vi "IO_Process.vi"(8 "error in":errorcluster, 10 "TopLevel":refnum<class "TopLevel.lvclass">, 11 "IO in":refnum<class "IO.lvclass">) -> (3 "IO out":refnum<class "IO.lvclass">)   [LabVIEW 2022 SP3, in "IO.lvclass"]
uses:
  IO.lvclass
  TopLevel/TopLevel.lvclass
  TopLevel/Typedefs/Digilens Config Cluster.ctl
  TopLevel/Typedefs/Motor Controller Config Data.ctl
  Typedefs/IO Config Data.ctl
  Typedefs/DCON_DeviceConfig--Cluster.ctl
  Typedefs/Channel Data.ctl
  GIS Printer/Typedefs/PrinterConfiguration--Cluster.ctl
  DAQWFE/LV_Source/Subsystems/DAQ/DataTypes/TD DAQ Settings--cluster.ctl
  DAQWFE/LV_Source/Subsystems/DAQ/DataTypes/TD DI Instrument Settings--cluster.ctl
  DAQWFE/LV_Source/Subsystems/DAQ/DataTypes/TD AI Instrument Settings--cluster.ctl
  DAQWFE/LV_Source/Subsystems/DAQ/DataTypes/TD AI InstSettings--cluster.ctl
  DAQWFE/LV_Source/Subsystems/DAQ/Process/ProcessSupport/TD SimAI Ranges--cluster.ctl
  Typedefs/ReadbackQuery--Cluster.ctl
  Typedefs/Device Names.ctl
  Typedefs/DCON Action Engine-States.ctl
  Typedefs/DO Value API Data.ctl
  Typedefs/AO Value API Data.ctl
  Typedefs/API Event Data.ctl
  Typedefs/API Task State.ctl
  Typedefs/API Command Cluster.ctl
  Typedefs/API Command Enum.ctl
  Typedefs/Purge PH API Data.ctl
  Typedefs/ICP1-D0 Channel Names.ctl
  Typedefs/ICP2-DI Channel Names.ctl
  Typedefs/ICP2-DO Channel Names.ctl
  Typedefs/ICP1-AI Channel Names.ctl
  Typedefs/ICP1-AO Channel Names.ctl
  Typedefs/ICP2-AO Channel Names.ctl
  Motor Controller/Motor Controller.lvclass
  GIS Printer/GIS Printer.lvclass
  DAQWFE/LV_Source/Subsystems/DAQ/DAQ.lvclass
panel:
  out "error out":errorcluster
  in  "OK":bool
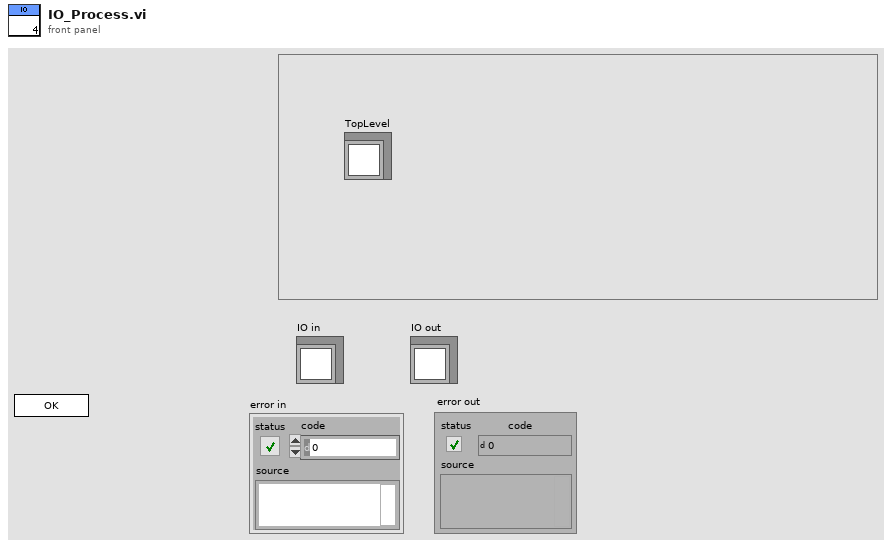
[diagram p1: front panel]
types:
  T1 = typedef "ReadbackQuery--Cluster.ctl" = cluster{"Device Name":T2, "Action":T3}
  T2 = typedef "IO.lvclass/Device Names.ctl" = enum16{"ICP1-DO", "ICP2-DI", "ICP2-DO", "ICP1-AI", "ICP1-AO", "ICP2-AO"}
  T3 = typedef "DCON Action Engine-States.ctl" = enum16{"Open", "Close", "Set DO Value", "Get Digital Status", "Get Data", "Get AI Status", "Set AO Value", "Get AO Status"}
  T4 = typedef "TopLevel.lvclass/Digilens Config Cluster.ctl" = cluster{"Motion Controller":T5, "IO Config":T6, "PrinterConfiguration":T9, "DAQ Settings":T10}
  T5 = typedef "Motor Controller.lvclass/Motor Controller Config Data.ctl" = cluster{"Motor IP Addresss":string, "Current Position":i32, "Pulse_Per_mm":i32, "PrePrint":dbl[], "Load Position_mm":i32, "Laminate Position_mm":i32}
  T6 = typedef "IO.lvclass/IO Config Data.ctl" = cluster{"DAQDevices":T7[], "DI Channels":T8[], "DO Channels":T8[], "Material Names":string[], "AI Channels":T8[], "AO Channels":T8[]}
  T7 = typedef "IO.lvclass/DCON_DeviceConfig--Cluster.ctl" = cluster{"COM":string, "DeviceName":string, "BaudRate":u32, "Number of Channels":i32, "DeviceAddress":i32, "Enable":bool}
  T8 = typedef "IO.lvclass/Channel Data.ctl" = cluster{"Channel Name":string, "Device Name":string, "Channel No":string}
  T9 = typedef "GIS Printer.lvclass/PrinterConfiguration--Cluster.ctl" = cluster{"IPAddress":string, "Move Stage on RTP Command?":bool, "Stage Move Position":string, "PH1-Prime Path":path, "PH2-Prime Path":path, "PH3-Prime Path":path, "PH4-Prime Path":path, "PH5-Prime Path":path, "PH6-Prime Path":path, "PrintScriptsFolder":path, "PurgeScriptsFolder":path, "StageScriptsFolder":path, "PH1-HeatOn Path":path, "PH2-HeatOn Path":path, "PH3-HeatOn Path":path, "PH4-HeatOn Path":path, "PH5-HeatOn Path":path, "PH6-HeatOn Path":path, "PH1-HeatOff Path":path, "PH2-HeatOff Path":path, "PH3-HeatOff Path":path, "PH4-HeatOff Path":path, "PH5-HeatOff Path":path, "PH6-HeatOff Path":path}
  T10 = typedef "DAQ.lvclass/TD DAQ Settings--cluster.ctl" = cluster{"Simulate DAQ":bool, "DI Settings":T11[], "AI Settings":T12[], "Relay IONames":string[], "AO IONames":string[], "AO NChan SingleTask":bool}
  T11 = typedef "DAQ.lvclass/TD DI Instrument Settings--cluster.ctl" = cluster{"Disable":bool, "DI TaskName":string, "DI RefreshIntv":i32}
  T12 = typedef "DAQ.lvclass/TD AI Instrument Settings--cluster.ctl" = cluster{"Disable":bool, "AI TaskName":string, "AI InstSettings":T13, "SimAI Ranges":T14}
  T13 = typedef "DAQ.lvclass/TD AI InstSettings--cluster.ctl" = cluster{"DaqRate":dbl, "NumSamples":i32}
  T14 = typedef "DAQ.lvclass/TD SimAI Ranges--cluster.ctl" = cluster{"lo":dbl, "hi":dbl}
  T15 = cluster{"IOLoopEvents":refnum<user-event>, "Open":bool, "Digilens Config":T4}
  T16 = typedef "IO.lvclass/API Event Data.ctl" = cluster{"Task":cluster{"Time Stamp":timestamp, "Timeout (ms)":u32, "Task State":T17, "Task Error":errorcluster, "Task ID":string}, "Command":variant, "Return Value":variant}
  T17 = typedef "IO.lvclass/API Task State.ctl" = enum16{"Completed", "Errored", "Pending"}
  T18 = typedef "IO.lvclass/API Command Cluster.ctl" = cluster{"Command":T19, "Arguments":string, "Data":variant}
  T19 = typedef "IO.lvclass/API Command Enum.ctl" = enum16{"Set DO Value", "Set AO Value", "Purge PH"}
  T20 = enum32{"invalid app kind", "Development System", "Run Time System", "Student Edition", "Embedded LabVIEW", "Evaluation", "Custom"}
  T21 = enum32{"Invalid", "Standard", "Closed", "Hidden", "Minimized", "Maximized"}
  T22 = typedef "IO.lvclass/DO Value API Data.ctl" = cluster{"Device Name":T2, "Value":bool, "Index":i32}
  T23 = typedef "IO.lvclass/AO Value API Data.ctl" = cluster{"Device Name":T2, "Index":i32, "Value":dbl}
  T24 = typedef "IO.lvclass/Purge PH API Data.ctl" = cluster{"ICP1-DO Channel Name":T25, "Duration (s)":dbl}
  T25 = typedef "IO.lvclass/ICP1-D0 Channel Names.ctl" = enum16{"None", "Meniscus Pressure Reg PWR - R1", "Meniscus Pressure Reg PWR - R2", "Meniscus Pressure Reg PWR - R3", "Meniscus Pressure Reg PWR - R4", "Meniscus Pressure Reg PWR - R5", "Meniscus Pressure Reg PWR - R6", "Clear Stage Alarm", "Servo ON", "Purge Valve Open - R1", "Purge Valve Open - R2", "Purge Valve Open - R3", "Purge Valve Open - R4", "Purge Valve Open - R5", "Purge Valve Open - R6"}
  T26 = typedef "IO.lvclass/ICP2-DI Channel Names.ctl" = enum16{"None", "SW - Ink Valve - R1", "SW - Ink Valve - R2", "SW - Ink Valve - R3", "SW - Ink Valve - R4", "SW - Ink Valve - R5", "SW - Ink Valve - R6", "SW - COVER INPUT SIDE", "SW - COVER OUTPUT SIDE", "SW - Purge - R1", "SW - Purge - R2", "SW - Purge - R3", "SW - Purge - R4", "SW - Purge - R5", "SW - Purge - R6"}
  T27 = typedef "IO.lvclass/ICP2-DO Channel Names.ctl" = enum16{"None", "Meniscus Valve Open - R1", "Meniscus Valve Open - R2", "Meniscus Valve Open - R3", "Meniscus Valve Open - R4", "Meniscus Valve Open - R5", "Meniscus Valve Open - R6", "Ink Flow Valve Open - R1", "Ink Flow Valve Open - R2", "Ink Flow Valve Open - R3", "Ink Flow Valve Open - R4", "Ink Flow Valve Open - R5", "Ink Flow Valve Open - R6", "SW_LED - Ink Valve - R1", "SW_LED - Ink Valve - R2", "SW_LED - Ink Valve - R3", "Recirc Pump On - R1", "Recirc Pump On - R2", "Recirc Pump On - R3", "Recirc Pump On - R4", "Recirc Pump On - R5", "Recirc Pump On - R6", "SW_LED - Ink Valve - R4", "SW_LED - Ink Valve - R5", "SW_LED - Ink Valve - R6"}
  T28 = typedef "IO.lvclass/ICP1-AI Channel Names.ctl" = enum16{"None", "Meniscus Pressure Read - R1", "Meniscus Pressure Read - R2", "Meniscus Pressure Read - R3", "Meniscus Pressure Read - R4", "Meniscus Pressure Read - R5", "Meniscus Pressure Read - R6", "Meniscus Pressure Set - R1", "Meniscus Pressure Set - R2", "Meniscus Pressure Set - R3", "Meniscus Pressure Set - R4", "Meniscus Pressure Set - R5", "Meniscus Pressure Set - R6"}
  T29 = typedef "IO.lvclass/ICP1-AO Channel Names.ctl" = enum16{"None", "Meniscus Pressure Set - R1", "Meniscus Pressure Set - R2", "Meniscus Pressure Set - R3", "Meniscus Pressure Set - R4", "Meniscus Pressure Set - R5", "Meniscus Pressure Set - R6", "Meniscus Vac Pump Speed"}
  T30 = typedef "IO.lvclass/ICP2-AO Channel Names.ctl" = enum16{"None", "Recirc Pump Flow Set - R1", "Recirc Pump Flow Set - R2", "Recirc Pump Flow Set - R3", "Recirc Pump Flow Set - R4", "Recirc Pump Flow Set - R5", "Recirc Pump Flow Set - R6"}
  T31 = cluster{"Time Stamp":timestamp, "Timeout (ms)":u32, "Task State":T17, "Task Error":errorcluster, "Task ID":string}
  T32 = cluster{"Core":cluster{"Current VI Reference":refnum<vi>, "Close Panel on Exit?":bool}, "TopLevel out":refnum<class "IO.lvclass">, "Tasks":T16[], "TO":i32, "API Executed Event":refnum<user-event>, "API Return Event":refnum<user-event>, "Task Start ms":u32, "Current Task. Return Value":variant, "Methods:Accessors:Digilens Config":T4, "Current Task":T18, "DCONOpen":bool}
  T33 = cluster{"Current VI Reference":refnum<vi>, "Close Panel on Exit?":bool}
  T34 = typedef "IO.lvclass/UserEvents.ctl" = cluster{"API Incoming Event":refnum<user-event>, "API Executed Event":refnum<user-event>, "API Return Event":refnum<user-event>, "Status Changed Event":refnum<user-event>}
  T35 = typedef "TopLevel.lvclass/UserEvents.ctl" = cluster{"API Incoming Event":refnum<user-event>, "API Executed Event":refnum<user-event>, "API Return Event":refnum<user-event>, "Exit Event":refnum<user-event>, "StatusChanged":refnum<user-event>, "DLP GUI Config Changed":refnum<user-event>, "AppEvent":refnum<user-event>, "Login Event":refnum<user-event>, "HeadPrimeStatusEvent":refnum<user-event>}
  T36 = typedef "IO.lvclass/DCON Private Data.ctl" = cluster{"DeviceName":string, "Number of Channels":i32, "COM":refnum<visa-resource-name>, "Status String":string, "Input String":string, "Value ":i32, "Digital Bits Value":bool[], "Analog Values":dbl[], "DeviceAddress":i32, "Enable":bool}
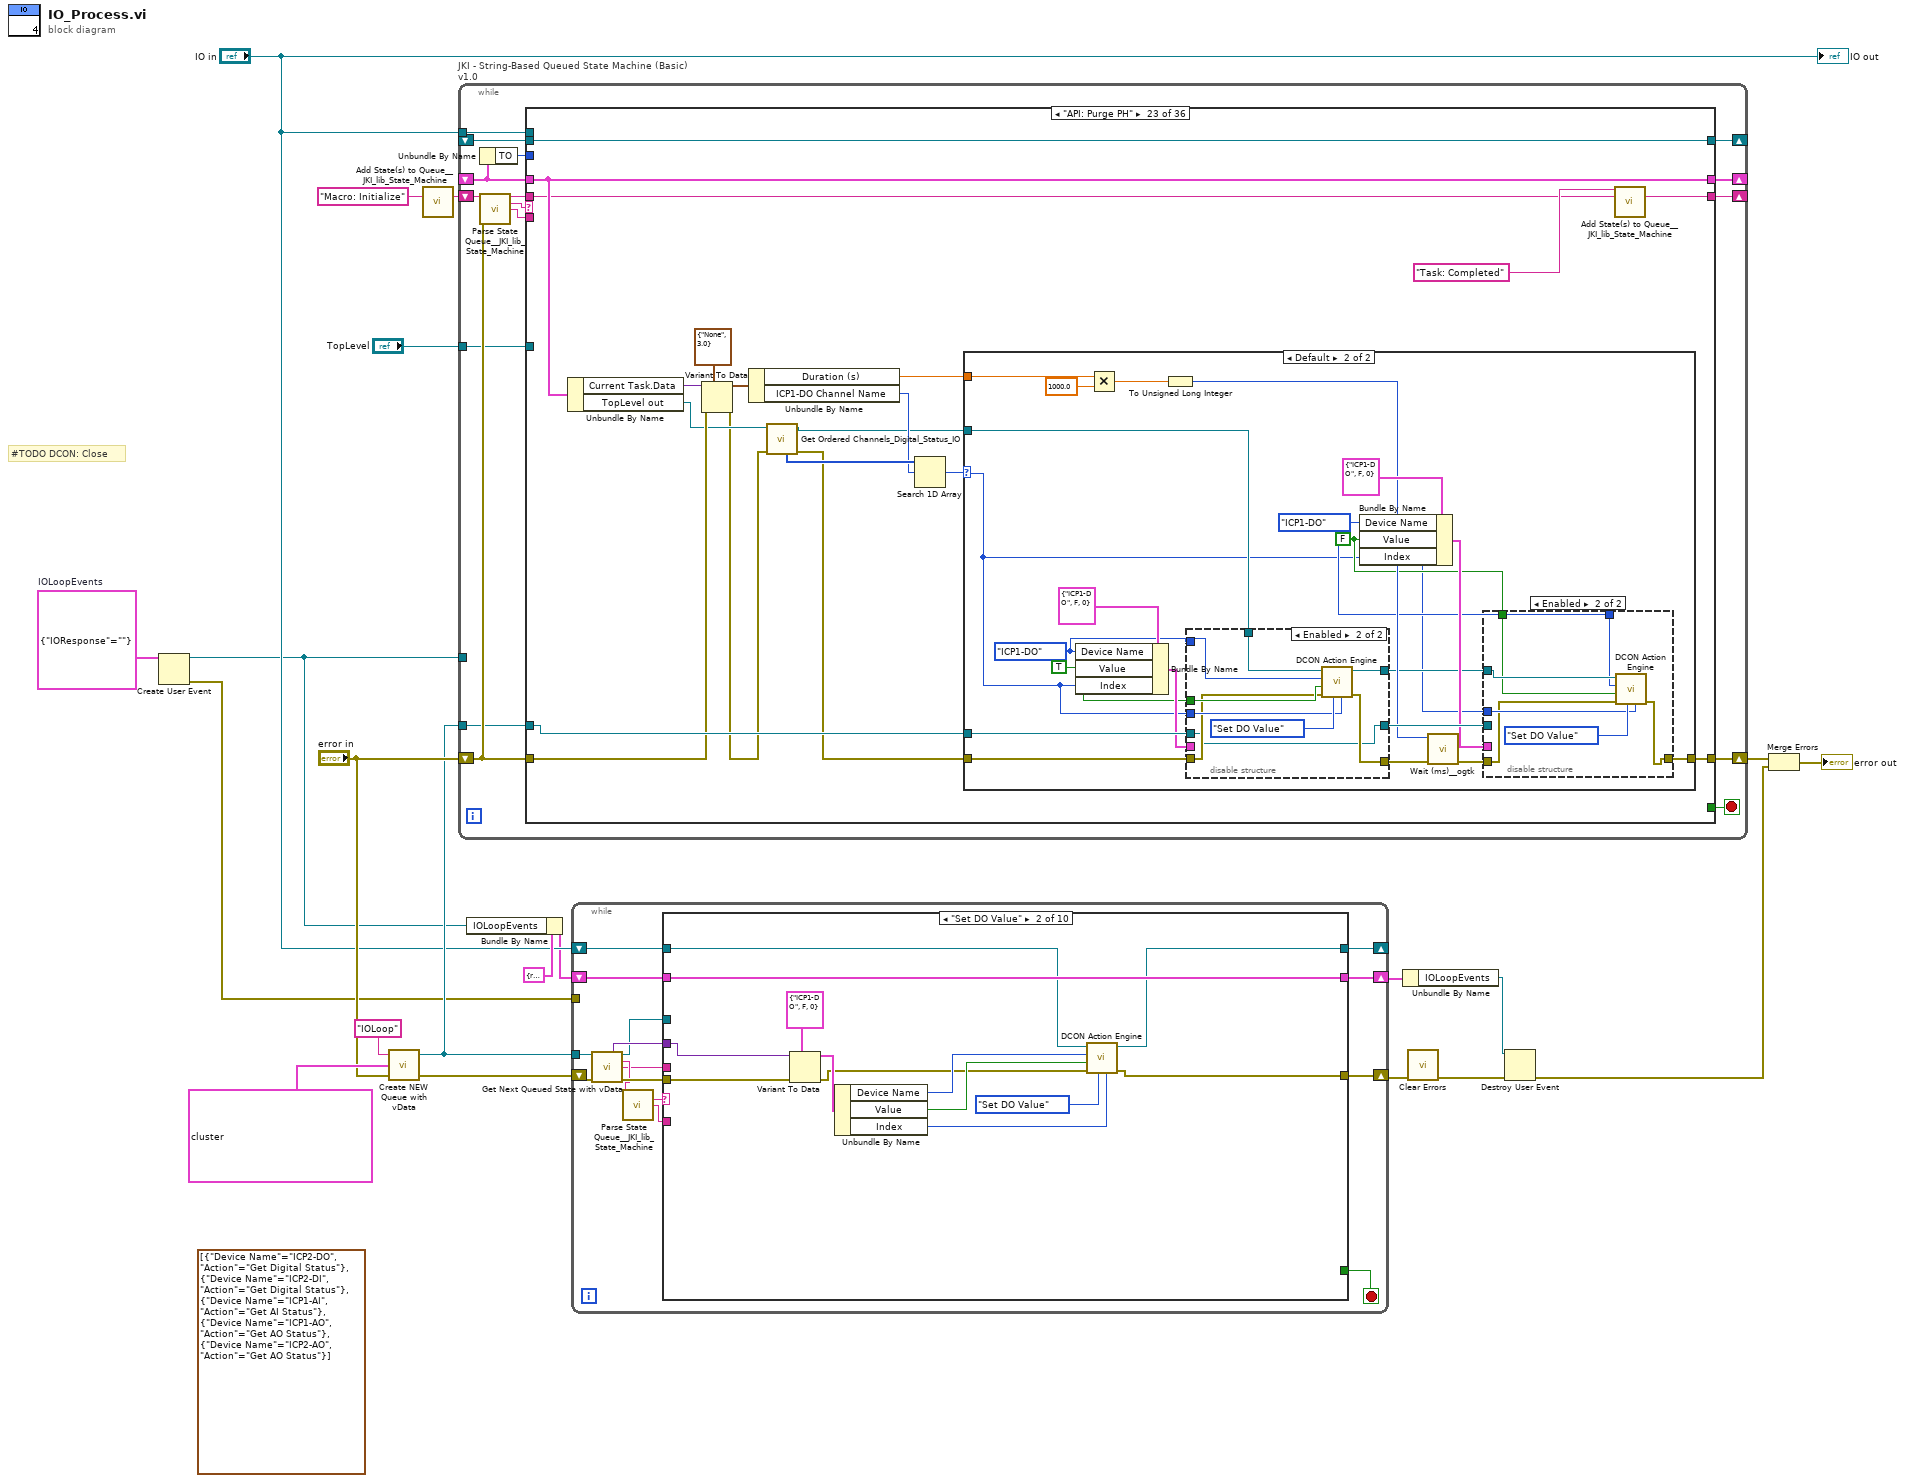
[diagram p0: block diagram]
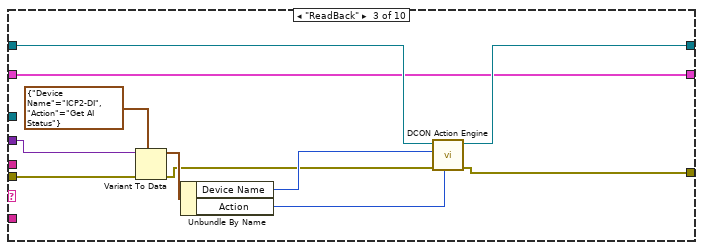
[diagram p3: hidden frame]
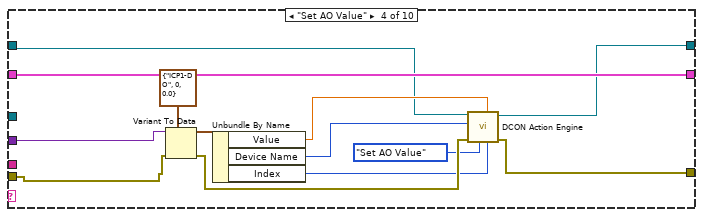
[diagram p4: hidden frame]
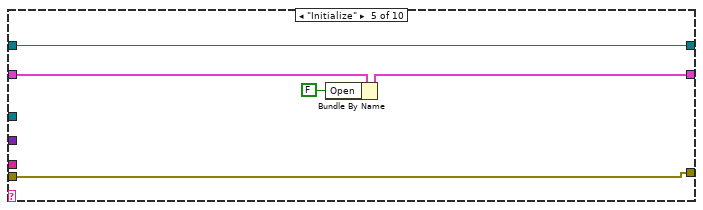
[diagram p5: hidden frame]
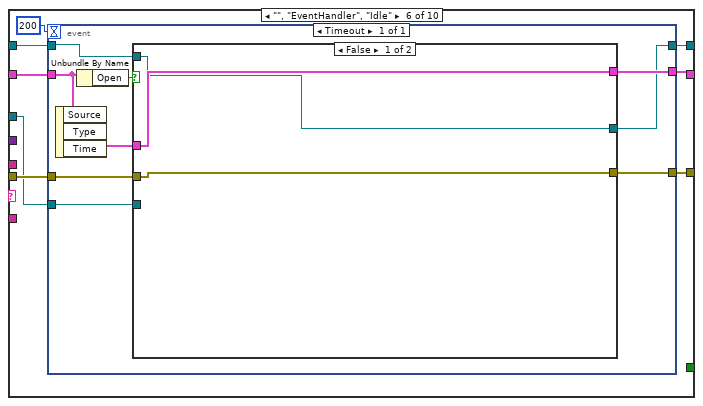
[diagram p6: hidden frame]
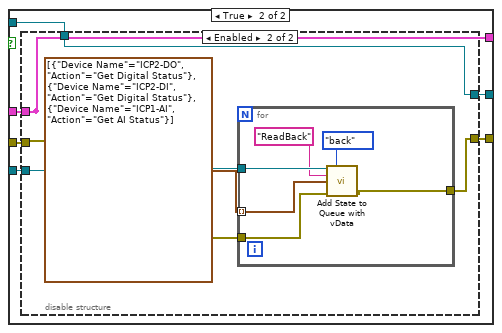
[diagram p7: hidden frame]
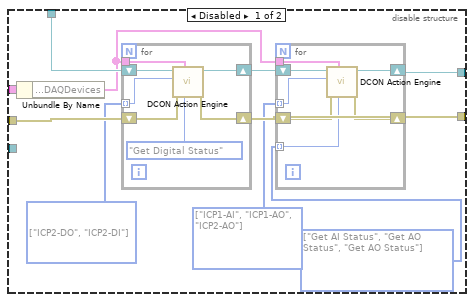
[diagram p8: hidden frame]
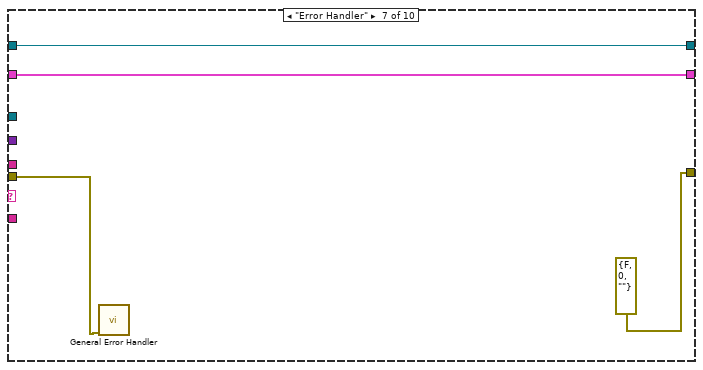
[diagram p9: hidden frame]
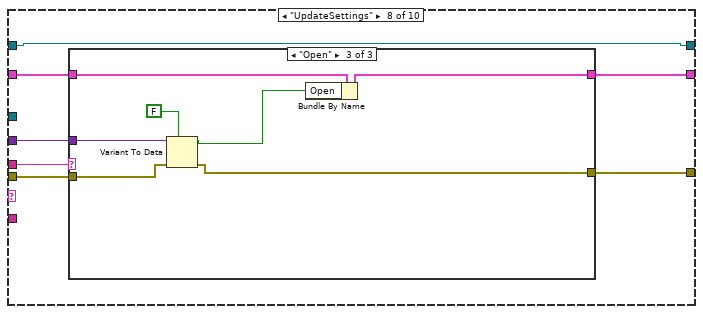
[diagram p10: hidden frame]
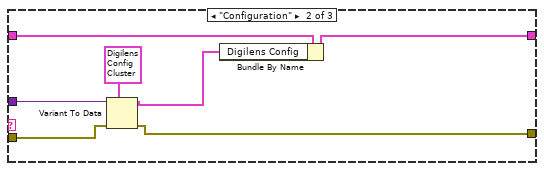
[diagram p12: hidden frame]
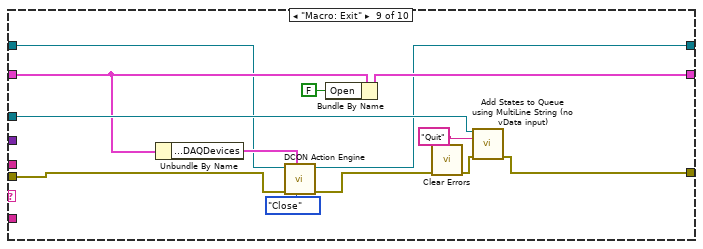
[diagram p13: hidden frame]
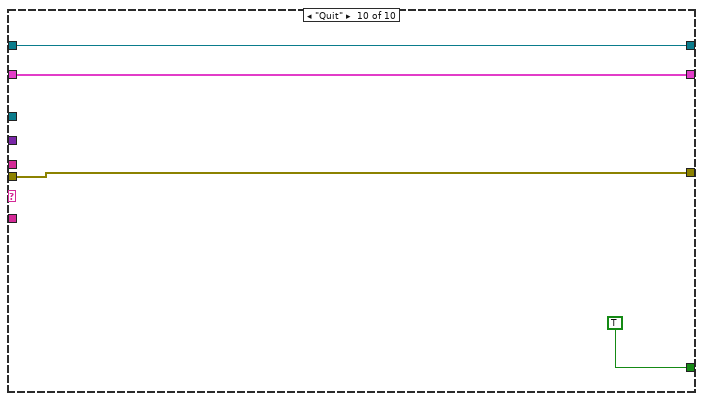
[diagram p14: hidden frame]
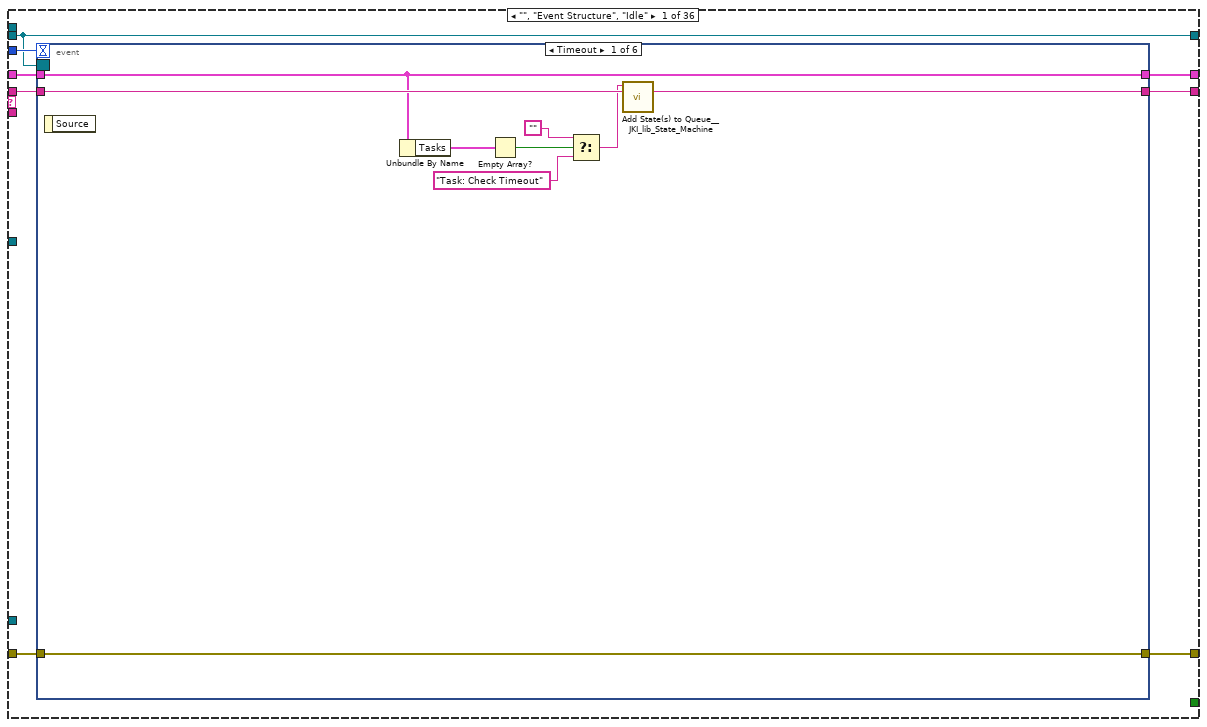
[diagram p15: hidden frame]
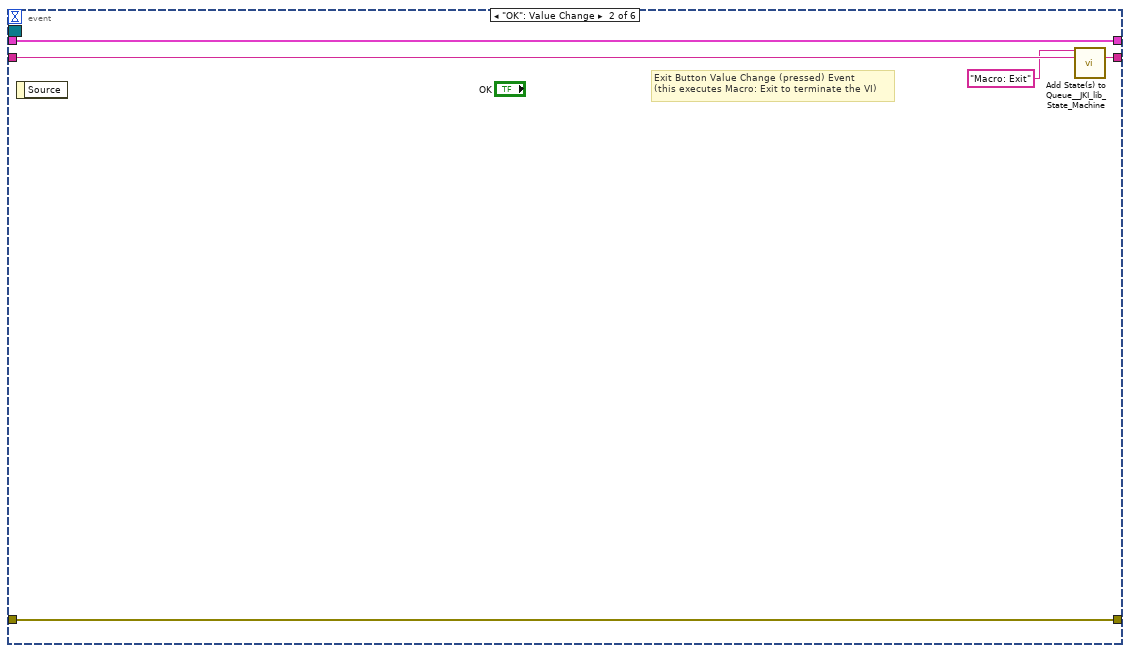
[diagram p16: hidden frame]
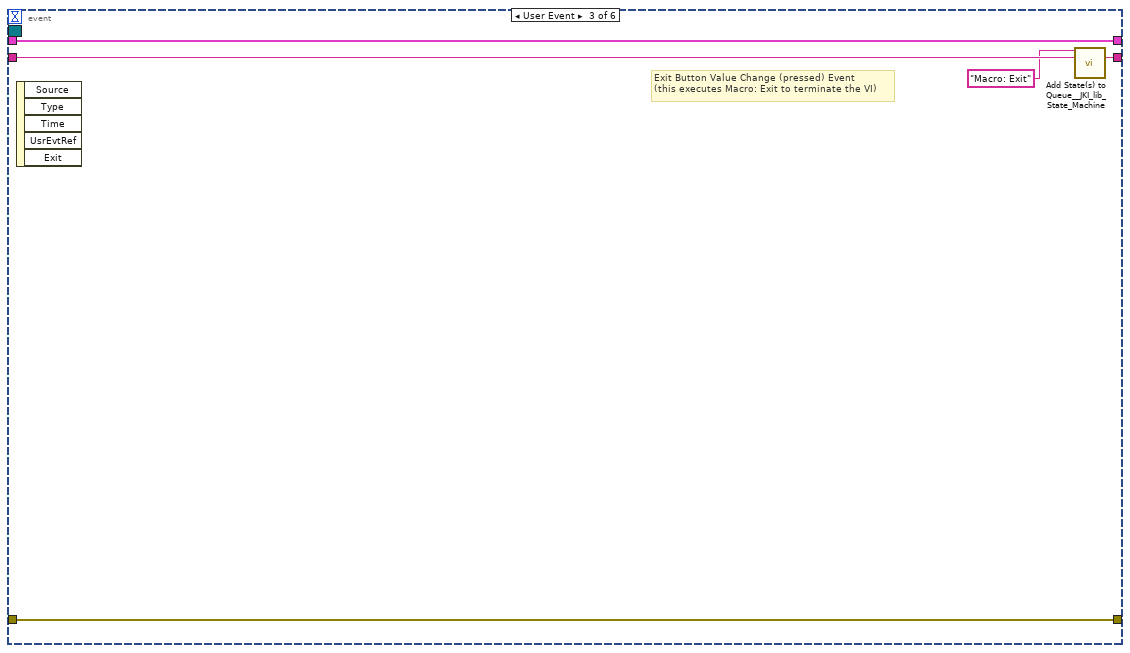
[diagram p17: hidden frame]
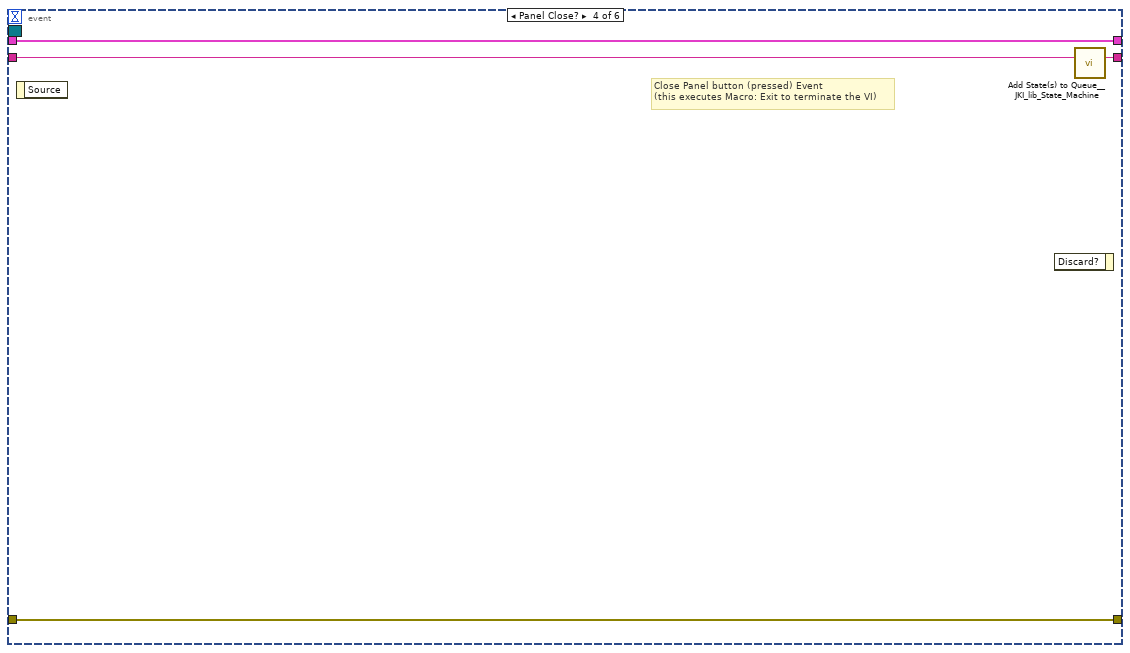
[diagram p18: hidden frame]
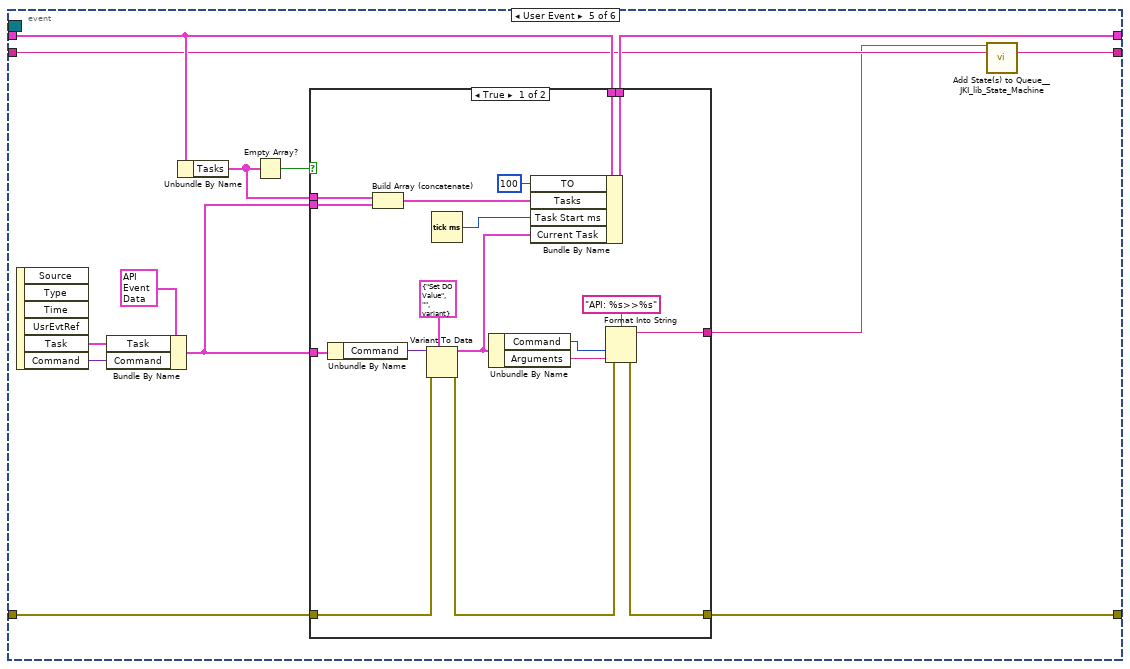
[diagram p19: hidden frame]
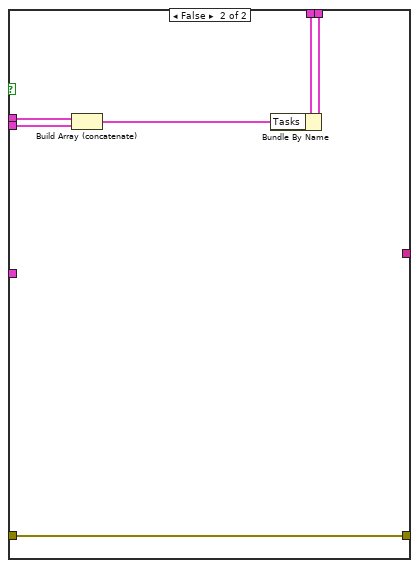
[diagram p20: hidden frame]
diagram:
  (unwired) T1[] [{"Device Name"=enum."ICP2-DO", "Action"=enum."Get Digital Status"}, {"Device Name"=enum."ICP2-DI", "Action"=enum."Get Digital Status"}, {"Device Name"=enum."ICP1-AI", "Action"=enum."Get AI Status"}, {"Device Name"=enum."ICP1-AO", "Action"=enum."Get AO Status"}, {"Device Name"=enum."ICP2-AO", "Action"=enum."Get AO Status"}]
  w17 = cluster{"IOResponse":string} {"IOResponse"=""}  # IOLoopEvents
  # "#TODO DCON: Close"
  n1 = Create User Event(user event datatype=w17) -> (user event=w5:refnum<user-event>, error out=w8:errorcluster)  [unwired: 1 in]
  n2 = call <vilib>:"Create NEW Queue with vData.vi"("error in (no error)"="error in", "Initial States"=cluster{"state":string, "vData":variant}[] [{"state"="Initialize", "vData"=variant}, {"state"="Idle", "vData"=variant}], "Name (SMQ)"="IOLoop") -> ("error out"=w12:errorcluster, "queue out"=w11:refnum<queue>)  [unwired: 1 in]
  n3 = call <vilib>:"Add State(s) to Queue__JKI_lib_State_Machine.vi"("State(s) in (\"\")"="Macro: Initialize") -> ("States Out"=w21:string)  [unwired: 14 in]
  n4 = while "JKI - String-Based Queued State Machine (Basic) v1.0" {
    shift-right: [w30] -> _
    shift-left: _ -> [w24]
    shift-right: [w33] -> w19
    shift-left: "error in" -> [w29]
    shift-right: [w32] -> _
    shift-left: w21 -> [w34]
    tunnel: "IO in" -> [w28]
    shift-right: [w27] -> _
    shift-left: _ -> [w26]
    tunnel: "TopLevel" -> [w23]
    tunnel: w5 -> [_]
    tunnel: w11 -> [w22]
    stop <- w31 stop-if-true
    n5 = Unbundle By Name(w24) -> ("TO"=w25:i32)
    n6 = call <vilib>:"Parse State Queue__JKI_lib_State_Machine.vi"("State Queue"=w34, "Error In (no error)"=w29) -> ("Remaining States"=w36:string, "Current State"=w37:string, "Arguments"=w35:string)  [unwired: 11 in]
    n7 = case shown="\"API: Purge PH\"" w37 {
      selector: w37 -> [_ _ w148 _ _ _ _ _ _ _ _ _ _ _ _ _ _ _ _ _ _ _ _ _ _ _ _ _ _ _ _ _ _ _ _ _]
      tunnel: w36 -> [w45 w146 w152 w171 w178 w184 w189 w213 w220 w225 w231 w238 w250 w277 _ w298 w309 w323 w329 w331 w339 w370 w403 w460 w471 w490 w511 w546 w558 w571 w583 w627 w671 w715 w759 w803]
      tunnel: w35 -> [_ _ _ _ _ _ _ _ _ _ _ w233 w244 _ _ _ _ _ _ _ _ _ _ _ _ _ _ _ _ _ _ _ _ _ _ _]
      tunnel: w24 -> [w43 w143 w150 w162 w175 w182 w186 _ w215 w222 w229 w236 w246 w274 w279 w296 w307 w320 w327 w332 w343 w375 w406 w461 w469 w488 w508 w543 w557 w569 w581 w625 w669 w713 w757 w801]
      tunnel: [w42 w144 w154 w168 errorcluster {"status"=FALSE, "code"=0, "source"=""} ("error out") w181 w187 w195 w216 w223 w226 w234 w247 w275 w282 w288 w308 w318 w326 w330 w335 w367 w402 w459 w465 w485 w516 w542 w559 w564 w579 w623 w667 w711 w755 w799] -> w33
      tunnel: w29 -> [w41 w144 w153 w168 w174 w181 w187 w206 w217 w223 w227 w235 w248 w275 w282 w283 w308 w311 w325 w330 w342 w374 w396 w459 w464 w484 w515 w541 w559 w567 w578 w622 w666 w710 w754 w798]
      tunnel: [w44 w145 w151 w170 w177 w183 w188 w212 w219 w224 w230 w237 w249 w276 w281 w297 w309 w322 w328 w331 w340 w371 w404 w460 w471 w490 w512 w547 w558 w571 w583 w627 w671 w715 w759 w803] -> w32
      tunnel: [_ _ _ _ _ TRUE _ _ _ _ _ _ _ _ _ _ _ _ _ _ _ _ _ _ _ _ _ _ _ _ _ _ _ _ _ _] -> w31
      tunnel: [w40 w143 w150 w169 w175 w182 w186 w211 w215 w222 w229 w236 w246 w274 w279 w296 w307 w320 w327 w332 w343 w375 w406 w461 w469 w488 w509 w540 w557 w562 w581 w625 w669 w713 w757 w801] -> w30
      tunnel: w25 -> [w39 _ _ _ _ _ _ _ _ _ _ _ _ _ _ _ _ _ _ _ _ _ _ _ _ _ _ _ _ _ _ _ _ _ _ _]
      tunnel: w28 -> [_ _ _ _ _ _ _ w191 _ _ _ _ _ _ _ _ _ _ _ _ _ _ _ _ _ _ _ _ _ _ _ _ _ _ _ _]
      tunnel: [w38 w142 w147 w159 w172 w179 w185 w209 w214 w221 w228 w232 w243 w273 w278 w293 w306 w321 w324 w333 w344 w376 w407 w462 w470 w489 w519 w548 w556 w570 w582 w626 w670 w714 w758 w802] -> w27
      tunnel: w26 -> [w38 w142 w147 w159 w172 w179 w185 w209 w214 w221 w228 w232 w243 w273 w278 w293 w306 _ w324 w333 w344 w376 w407 w462 w470 w489 w519 w548 w556 w570 w582 w626 w670 w714 w758 w802]
      tunnel: w23 -> [_ _ _ _ _ _ _ w200 _ _ _ _ _ _ _ _ _ w313 _ _ _ _ _ _ _ _ _ _ _ _ _ _ _ _ _ _]
      tunnel: w22 -> [_ _ _ _ _ _ _ w193 _ _ _ _ _ _ _ w285 _ _ _ _ w337 w366 w401 _ _ _ _ _ _ w563 _ _ _ _ _ _]
      frame "", "Event Structure", "Idle" {
        n8 = event shown="[0] Timeout" {
          selector: w38 -> [_ _ _ _ _ _]
          dyn-events: _ -> [_ _ _ _ _ _]
          timeout: w39 -> [_ _ _ _ _ _]
          tunnel: w45 -> [w54 w59 w64 w68 w70 w125]
          tunnel: [w53 w58 w63 w67 w71 w126] -> w44
          tunnel: w43 -> [w51 w56 w61 w65 w75 w124]
          tunnel: [w52 w57 w62 w66 w73 w118] -> w42
          tunnel: w41 -> [w52 w57 w62 w66 w72 w119]
          tunnel: [w51 w56 w61 w65 w76 w121] -> w40
          event Timeout {
            n9 = event-data() -> ()  [unwired: 1 in, 1 out]
            n10 = Unbundle By Name(w51) -> ("Tasks"=w50:T16[])
            n11 = Empty Array?(array=w50) -> (empty?=w49:bool)
            n12 = Select(t="", s=w49, f="Task: Check Timeout") -> (s? t:f=w46:string)
            n13 = call <vilib>:"Add State(s) to Queue__JKI_lib_State_Machine.vi"("State(s) in Front (\"\")"=w46, "State(s) in (\"\")"=w54) -> ("States Out"=w53:string)  [unwired: 13 in]
          }
          event "OK": Value Change {
            # "Exit Button Value Change (pressed) Event\n(this executes Macro: Exit to terminate the VI)"
            n14 = event-data() -> ()  [unwired: 1 in, 1 out]
            n15 = call <vilib>:"Add State(s) to Queue__JKI_lib_State_Machine.vi"("State(s) in Front (\"\")"="Macro: Exit", "State(s) in (\"\")"=w59) -> ("States Out"=w58:string)  [unwired: 13 in]
          }
          event User Event {
            # "Exit Button Value Change (pressed) Event\n(this executes Macro: Exit to terminate the VI)"
            n16 = event-data() -> ()  [unwired: 1 in, 5 out]
            n17 = call <vilib>:"Add State(s) to Queue__JKI_lib_State_Machine.vi"("State(s) in Front (\"\")"="Macro: Exit", "State(s) in (\"\")"=w64) -> ("States Out"=w63:string)  [unwired: 13 in]
          }
          event Panel Close? {
            # "Close Panel button (pressed) Event\n(this executes Macro: Exit to terminate the VI)"
            n18 = event-data() -> ()  [unwired: 1 in, 1 out]
            n19 = event-data() -> ()  [unwired: 2 in, 1 out]
            n20 = call <vilib>:"Add State(s) to Queue__JKI_lib_State_Machine.vi"("State(s) in (\"\")"=w68) -> ("States Out"=w67:string)  [unwired: 14 in]
          }
          event User Event {
            n21 = event-data() -> ("Task"=w80:T31, "Command"=w79:variant)  [unwired: 1 in, 4 out]
            n22 = Bundle By Name(cluster=T16 {"Task"={"Time Stamp"=timestamp(0 s since 1904-01-01), "Timeout (ms)"=0, "Task State"=enum."Completed", "Task Error"={"status"=FALSE, "code"=0, "source"=""}, "Task ID"=""}, "Command"=variant, "Return Value"=variant} ("API Event Data"), "Task"=w80, "Command"=w79) -> (w74:T16)
            n23 = Unbundle By Name(w75) -> ("Tasks"=w77:T16[])
            n24 = Empty Array?(array=w77) -> (empty?=w78:bool)
            n25 = case shown="True" w78 {
              tunnel: w77 -> [w99 w105]
              tunnel: w74 -> [w98 w104]
              tunnel: w75 -> [w97 w103]
              tunnel: [w95 w101] -> w76
              tunnel: w74 -> [w94 _]
              tunnel: w72 -> [w91 w100]
              tunnel: [w89 w100] -> w73
              tunnel: [w86 _] -> w69
              frame True {
                n26 = Unbundle By Name(w94) -> ("Command"=w93:variant)
                n27 = Build Array (concatenate)(w99, w98) -> (w96:T16[])
                n28 = Variant To Data(error in=w91, type=T18 {"Command"=enum."Set DO Value", "Arguments"="", "Data"=variant} ("API Command Cluster"), Variant=w93) -> (data=w82:T18, error out=w90:errorcluster)
                n29 = Tick Count (ms)() -> (millisecond timer value=w84:u32)
                n30 = Unbundle By Name(w82) -> ("Command"=w87:T19, "Arguments"=w85:string)
                n31 = Bundle By Name(cluster=w97, "TO"=100, "Tasks"=w96, "Task Start ms"=w84, "Current Task"=w82) -> (w95:T32)
                n32 = Format Into String(format string="API: %s>>%s", error in=w90, w87, w85) -> (resulting string=w86:string, error out=w89:errorcluster)  [unwired: 1 in]
              }
              frame False {
                n33 = Build Array (concatenate)(w105, w104) -> (w102:T16[])
                n34 = Bundle By Name(cluster=w103, "Tasks"=w102) -> (w101:T32)
              }
            }
            n35 = call <vilib>:"Add State(s) to Queue__JKI_lib_State_Machine.vi"("State(s) in Front (\"\")"=w69, "State(s) in (\"\")"=w70) -> ("States Out"=w71:string)  [unwired: 13 in]
          }
          event User Event {
            n36 = event-data() -> ("Task"=w112:T31, "Command"=w116:variant, "Return Value"=w115:variant)  [unwired: 1 in, 4 out]
            n37 = Unbundle By Name(w124) -> ("API Return Event"=w109:refnum<user-event>, "Tasks"=w123:T16[])
            n38 = Bundle By Name(cluster=T16 {"Task"={"Time Stamp"=timestamp(0 s since 1904-01-01), "Timeout (ms)"=0, "Task State"=enum."Completed", "Task Error"={"status"=FALSE, "code"=0, "source"=""}, "Task ID"=""}, "Command"=variant, "Return Value"=variant} ("API Event Data"), "Task"=w112, "Command"=w116, "Return Value"=w115) -> (w114:T16)
            n39 = Delete From Array(array=w123, index=0) -> (deleted portion=w113:T16, array with subset deleted=w120:T16[])  [unwired: 1 in]
            n40 = Unbundle By Name(w113) -> ("Task.Task ID"=w111:string)
            n41 = Unbundle By Name(w112) -> ("Task ID"=w110:string, "Task State"=w107:T17)
            n42 = Equal?(x=w111, y=w110) -> (x = y?=w108:bool)
            n43 = case shown="True" w108 {
              tunnel: w124 -> [w128 w141]
              tunnel: [w128 w140] -> w121
              tunnel: w120 -> [_ w139]
              tunnel: w109 -> [_ w138]
              tunnel: w119 -> [w127 w135]
              tunnel: [w127 w136] -> w118
              tunnel: w114 -> [_ w137]
              tunnel: w107 -> [_ w134]
              tunnel: [_ w129] -> w106
              frame False {
              }
              frame True {
                n44 = Equal?(x=w134, y=API_Task_State."Errored") -> (x = y?=w132:bool)
                n45 = Select(t="Task: Remove on Error", s=w132, f="Task: Check Pending") -> (s? t:f=w129:string)
                n46 = Bundle By Name(cluster=w141, "Tasks"=w139) -> (w140:T32)
                n47 = Generate User Event(user event=w138, event data cluster=w137, error in=w135) -> (error out=w136:errorcluster)  [unwired: 1 in, 1 out]
              }
            }
            n48 = call <vilib>:"Add State(s) to Queue__JKI_lib_State_Machine.vi"("State(s) in Front (\"\")"=w106, "State(s) in (\"\")"=w125) -> ("States Out"=w126:string)  [unwired: 13 in]
          }
        }
      }
      frame "---------- Core ----------" {
        n49 = call <vilib>:"Add State(s) to Queue__JKI_lib_State_Machine.vi"("State(s) in (\"\")"=w146) -> ("States Out"=w145:string)  [unwired: 14 in]
      }
      frame Default {
        w157 = 42 items=["No error", "Argument error", "Memory is full", "Out of zone", "End of file", "File already open", "Generic file I/O error", "File not found", "File permission error", "Disk is full", "Duplicate path", "Too many files open", "System feature not enabled", "Resource file not found", "Cannot add resource", "Resource not found", "Image not found", "Image memory error", "Pen does not exist", "Config type invalid", "Config token not found", "Config parse error", "Config memory error", "Bad external code format", "Bad external code offset", "External code not present", "Null window", "Destroy window error", "Null menu", "Print aborted", "Bad print record", "Print driver error", "Windows error during printing", "Memory error during printing", "Print dialog error", "Generic print error", "Invalid device refnum", "Device not found", "Device parameter error", "Device unit error", "Cannot open device", "Device call aborted", "Generic error", "Cancelled by user", "Object ID too low", "Object ID too high", "Object not in heap", "Unknown heap", "Unknown object (invalid DefProc)", "Unknown object (DefProc not in table)", "Message out of range", "Invalid (null) method", "Unknown message", "Manager call not supported", "Bad address", "Network operation in progress", "Network operation timed out", "Connection is busy", "Network attribute not supported", "Network error", "Address in use", "System out of memory", "Connection aborted", "Connection refused", "Not connected", "Already connected", "Connection closed", "Initialization error (interapplication manager)", "Bad occurrence", "Wait on unbound occurrence handler", "Occurrence queue overflow", "Datalog type conflict", "Unused", "Unrecognized type (interapplication manager)", "Memory corrupt", "Failed to make temporary DLL", "Old CIN version", "Drag socket not found", "Failed to load drop-object", "Failed to register OLE object", "Failed to release OLE object", "Format specifier type mismatch", "Unknown format specifier", "Too few format specifiers", "Too many format specifiers", "Scan failed", "Newer CIN version", "Error converting to variant", "Runtime menu error", "Password tampered", "Variant attribute not found", "Incompatible variant data type", "Event data is not available", "Event Store is not present", "Occurrence is not found", "Event Queue is not created", "Event info is not available", "Refnum passed is NULL", "Error retrieving Class GUID", "Error retrieving CoClass GUID", "Error retrieving TypeLib GUID.", "Bad built application magic bytes.", "Specific driver is different from the specific driver associated with the Logical Name.", "There is no session opened to the class driver.", "Max Error", "MAX - Error with config objects", "MAX - Error loading configuration", "MAX - Group not supported"]
        # "Current State"
        # "Handle mistyped state name (developer tool)"
        n50 = Format Into String(format string="Software Exception: Unhandled State \"%s\"." ("message"), error in=w153, w148) -> (resulting string=w156:string, error out=w155:errorcluster)  [unwired: 1 in]
        n51 = call <vilib>:"Error Cluster From Error Code.vi"("show call chain? (False)"=TRUE, "error in (no error)"=w155, "error message (\"\")"=w156, "error code (0)"=w157) -> ("error out"=w154:errorcluster)  [unwired: 5 in]
        n52 = call <vilib>:"Add State(s) to Queue__JKI_lib_State_Machine.vi"("State(s) in (\"\")"=w152) -> ("States Out"=w151:string)  [unwired: 14 in]
      }
      frame "Initialize Core Data" {
        # "originally closed?"
        # "exe?"
        # "If panel starts closed or is an EXE, then close it when we exit"
        n53 = property class="VI"() -> ("Front Panel.Open"=w167:bool)  [unwired: 2 in, 2 out]
        n54 = property class="App"() -> ("App.Kind"=w166:T20)  [unwired: 2 in, 2 out]
        n55 = control-ref of="Current VI Reference"() -> (w160:refnum<vi>)
        n56 = Not(x=w167) -> (.not. x?=w164:bool)
        n57 = Equal?(x=w166, y=T20."Run Time System" ("Application:Kind")) -> (x = y?=w163:bool)
        n58 = Or(x=w164, y=w163) -> (x .or. y?=w161:bool)
        n59 = Bundle By Name(cluster=w162, "Core.Current VI Reference"=w160, "Core.Close Panel on Exit?"=w161) -> (w169:T32)
        n60 = call <vilib>:"Add State(s) to Queue__JKI_lib_State_Machine.vi"("State(s) in (\"\")"=w171) -> ("States Out"=w170:string)  [unwired: 14 in]
      }
      frame "Error Handler" {
        # "Unhandled Error -- Display it"
        # "Clear error"
        n61 = call <vilib>:"General Error Handler.vi"("error in (no error)"=w174) -> ()  [unwired: 10 in, 5 out]
        n62 = call <vilib>:"Add State(s) to Queue__JKI_lib_State_Machine.vi"("State(s) in Front (\"\")"="/* Post Error States", "State(s) in (\"\")"=w178) -> ("States Out"=w177:string)  [unwired: 13 in]
      }
      frame "Exit" {
        n63 = call <vilib>:"Add State(s) to Queue__JKI_lib_State_Machine.vi"("State(s) in (\"\")"=w184) -> ("States Out"=w183:string)  [unwired: 14 in]
      }
      frame "---------- Data ----------" {
        n64 = call <vilib>:"Add State(s) to Queue__JKI_lib_State_Machine.vi"("State(s) in (\"\")"=w189) -> ("States Out"=w188:string)  [unwired: 14 in]
      }
      frame "Data: Initialize" {
        w190 = FALSE  # DCONOpen
        w198 = T18 {"Command"=enum."Set DO Value", "Arguments"="", "Data"=variant}  # Current Task
        w201 = variant  # Current Task. Return Value
        w203 = u32 0  # Task Start ms
        w207 = -1  # TO
        w208 = T16[] []  # Tasks
        w210 = T33 {"Current VI Reference"=refnum, "Close Panel on Exit?"=FALSE}  # Core
        n65 = call-dynamic "GetEvents_IO.vi"("error in (no error)"=w206, "TopLevel in"=w191) -> ("error out"=w199:errorcluster, "UserEvents"=w205:T34, "TopLevel out"=w192:refnum<class "IO.lvclass">)  [unwired: 7 in]
        n66 = Unbundle By Name(w205) -> ("API Executed Event"=w204:refnum<user-event>, "API Return Event"=w202:refnum<user-event>)
        n67 = property class="TopLevel.lvclass"(reference=w200, error in=w199) -> (error out=w196:errorcluster, "Methods:Accessors:Digilens Config"=w194:T4)  [unwired: 1 out]
        n68 = call <vilib>:"Add State to Queue with vData.vi"("queue in"=w193, "state in"="UpdateSettings>>Configuration", "vData (\"\")"=w194, "error in"=w196) -> ("error out"=w195:errorcluster)  [unwired: 8 in, 3 out]
        n69 = Bundle("Core"=w210, "TopLevel out"=w192, "Tasks"=w208, "TO"=w207, "API Executed Event"=w204, "API Return Event"=w202, "Task Start ms"=w203, "Current Task. Return Value"=w201, "Methods:Accessors:Digilens Config"=w194, "Current Task"=w198, "DCONOpen"=w190) -> (w211:T32)  [unwired: 1 in]
        n70 = call <vilib>:"Add State(s) to Queue__JKI_lib_State_Machine.vi"("State(s) in (\"\")"=w213) -> ("States Out"=w212:string)  [unwired: 14 in]
      }
      frame "Data: Cleanup" {
        n71 = Unbundle By Name(w215) -> ("Core.Current VI Reference"=w218:refnum<vi>)
        n72 = Close Reference(reference=w218, error in (no error)=w217) -> (error out=w216:errorcluster)
        n73 = call <vilib>:"Add State(s) to Queue__JKI_lib_State_Machine.vi"("State(s) in (\"\")"=w220) -> ("States Out"=w219:string)  [unwired: 14 in]
      }
      frame "---------- UI ----------" {
        n74 = call <vilib>:"Add State(s) to Queue__JKI_lib_State_Machine.vi"("State(s) in (\"\")"=w225) -> ("States Out"=w224:string)  [unwired: 14 in]
      }
      frame "UI: Initialize" {
        n75 = call <userlib>:"Fit VI window to Largest Dec__ogtk.vi"("error in (no error)"=w227) -> ("error out"=w226:errorcluster)  [unwired: 5 in, 1 out]
        n76 = call <vilib>:"Add State(s) to Queue__JKI_lib_State_Machine.vi"("State(s) in (\"\")"=w231) -> ("States Out"=w230:string)  [unwired: 14 in]
      }
      frame "UI: Cursor Set" {
        # "Argument"
        n77 = case shown="\"Idle\", Default" w233 {
          tunnel: w235 -> [w240 w242]
          tunnel: [w239 w241] -> w234
          frame "Idle", Default {
            n78 = call <vilib>:"Unset Busy.vi"("error in (no error)"=w240) -> ("error out"=w239:errorcluster)  [unwired: 10 in]
          }
          frame "Busy" {
            n79 = call <vilib>:"Set Busy.vi"("error in (no error)"=w242) -> ("error out"=w241:errorcluster)  [unwired: 9 in, 1 out]
          }
        }
        n80 = call <vilib>:"Add State(s) to Queue__JKI_lib_State_Machine.vi"("State(s) in (\"\")"=w238) -> ("States Out"=w237:string)  [unwired: 14 in]
      }
      frame "UI: Front Panel State" {
        # "Argument"
        n81 = Unbundle By Name(w246) -> ("Core.Current VI Reference"=w245:refnum<vi>)
        n82 = case shown="\"Open\", Default" w244 {
          tunnel: w248 -> [w254 w267]
          tunnel: [w256 w268] -> w247
          tunnel: w245 -> [w255 w265]
          frame "Open", Default {
            n83 = property class="VI"(reference=w255, error in=w254) -> (reference out=w252:refnum<vi>, error out=w253:errorcluster, "Front Panel.Open"=w251:bool)
            n84 = case shown="False" w251 {
              tunnel: [w259 w262] -> w256
              tunnel: w253 -> [w258 w262]
              tunnel: w252 -> [w257 _]
              frame False {
                n85 = invoke class="VI" method="FP.Open"(reference=w257, error in=w258, "Activate"=TRUE, "State"=T21."Standard") -> (error out=w259:errorcluster)  [unwired: 1 in, 4 out]
              }
              frame True {
              }
            }
          }
          frame "Close" {
            n86 = property class="VI"(reference=w265, error in=w267) -> (reference out=w264:refnum<vi>, error out=w266:errorcluster, "Front Panel.Open"=w263:bool)
            n87 = case shown="True" w263 {
              tunnel: [w269 w272] -> w268
              tunnel: w266 -> [w269 w271]
              tunnel: w264 -> [_ w270]
              frame False {
              }
              frame True {
                n88 = invoke class="VI" method="FP.Close"(reference=w270, error in=w271) -> (error out=w272:errorcluster)  [unwired: 1 in, 2 out]
              }
            }
          }
        }
        n89 = call <vilib>:"Add State(s) to Queue__JKI_lib_State_Machine.vi"("State(s) in (\"\")"=w250) -> ("States Out"=w249:string)  [unwired: 14 in]
      }
      frame "---------- Macro ----------" {
        n90 = call <vilib>:"Add State(s) to Queue__JKI_lib_State_Machine.vi"("State(s) in (\"\")"=w277) -> ("States Out"=w276:string)  [unwired: 14 in]
      }
      frame "Macro: Initialize" {
        w280 = "Data: Initialize\nInitialize Core Data\nUI: Initialize\nEvents: Register Events\nInit: DCON Open\nInit: Set ICP1-DO Channels\nInit: Set ICP2-DI Channels\nInit: Set ICP2-DO Channels\nInit: Set ICP1-AI Channels\nInit: Set ICP1-AO Channels\nInit: Set ICP2-AO Channels\n/*UI: Front Panel State >> Open"  # Data: Initialize Initialize Core Data UI: Initialize Events: Register Events Init: DCON Open Init: Set ICP1-DO Channels Init: Set ICP2-DI Channels Init: Set ICP2-DO Channels Init: Set ICP1-AI Channels Init: Set ICP1-AO Channels Init: Set ICP2-AO Channels /*UI: Front Panel State >> Open
        n91 = call <vilib>:"Add State(s) to Queue__JKI_lib_State_Machine.vi"("State(s) in (\"\")"=w280) -> ("States Out"=w281:string)  [unwired: 14 in]
      }
      frame "Macro: Exit" {
        n92 = Flush Queue(queue=w285, error in (no error)=w283) -> (queue out=w286:refnum<queue>, error out=w284:errorcluster)  [unwired: 1 out]
        n93 = call <vilib>:"Add States to Queue using MultiLine String (no vData input).vi"("queue in"=w286, "mode (back)"=enum16{"back", "front"}."front", "states in"="Macro: Exit", "error in"=w284) -> ("error out"=w291:errorcluster)  [unwired: 9 in, 2 out]
        n94 = Unbundle By Name(w296) -> ("Core.Close Panel on Exit?"=w295:bool)
        n95 = call <userlib>:"Wait (ms)__ogtk.vi"("error in (no error)"=w291, "milliseconds to wait"=u32 2000) -> ("error out"=w289:errorcluster)  [unwired: 8 in, 1 out]
        n96 = flat-sequence {
          tunnel: w295 -> [w305]
          tunnel: [w300] -> w294
          tunnel: w289 -> [w299]
          tunnel: [w299] -> w288
          frame #0 {
            n97 = Select(t="UI: Front Panel State >> Close", s=w305, f="") -> (s? t:f=w302:string)
            n98 = call <vilib>:"Add State(s) to Queue__JKI_lib_State_Machine.vi"("State(s) in (\"\")"=w302, "State(s) at Back (\"\")"="Data: Cleanup\nEvents: Unregister Events\nExit") -> ("States Out"=w300:string)  [unwired: 13 in]
          }
        }
        n99 = call <vilib>:"Add State(s) to Queue__JKI_lib_State_Machine.vi"("State(s) in Front (\"\")"=w294, "State(s) in (\"\")"=w298) -> ("States Out"=w297:string)  [unwired: 13 in]
      }
      frame "---------- Events ----------" {
      }
      frame "Events: Register Events" {
        n100 = call-dynamic "GetEvents_TopLevel.vi"("error in (no error)"=w311, "TopLevel in"=w313) -> ("error out"=w312:errorcluster, "UserEvents"=w314:T35)  [unwired: 7 in, 1 out]
        n101 = Unbundle By Name(w314) -> ("Exit Event"=w310:refnum<user-event>)
        n102 = Unbundle By Name(w320) -> ("TopLevel out"=w319:refnum<class "IO.lvclass">)
        n103 = call-dynamic "GetEvents_IO.vi"("error in (no error)"=w312, "TopLevel in"=w319) -> ("error out"=w318:errorcluster, "UserEvents"=w317:T34)  [unwired: 7 in, 1 out]
        n104 = Unbundle By Name(w317) -> ("API Incoming Event"=w316:refnum<user-event>, "API Executed Event"=w315:refnum<user-event>)
        n105 = register-events(w316, w315, w310) -> (reference out=w321:refnum<event-registration>)  [unwired: 2 in, 1 out]
        n106 = call <vilib>:"Add State(s) to Queue__JKI_lib_State_Machine.vi"("State(s) in (\"\")"=w323) -> ("States Out"=w322:string)  [unwired: 14 in]
      }
      frame "Events: Unregister Events" {
        n107 = Unregister For Events(event registration refnum=w324, error in=w325) -> (error out=w326:errorcluster)
        n108 = call <vilib>:"Add State(s) to Queue__JKI_lib_State_Machine.vi"("State(s) in (\"\")"=w329) -> ("States Out"=w328:string)  [unwired: 14 in]
      }
      frame "---------- API ----------" {
      }
      frame "API: Set DO Value" {
        n109 = Unbundle By Name(w343) -> ("TopLevel out"=w341:refnum<class "IO.lvclass">, "Current Task.Data"=w336:variant)
        n110 = disable-structure shown="Disabled" {
          disable-tunnel: w342 -> [w362 w363]
          disable-tunnel: w341 -> [w361 _]
          disable-tunnel: [w360 w363] -> w334
          disable-tunnel: w336 -> [w352 _]
          frame Disabled {
            n111 = Variant To Data(error in=w362, type=T22 {"Device Name"=enum."ICP1-DO", "Value"=FALSE, "Index"=0} ("DO Value Input"), Variant=w352) -> (data=w357:T22, error out=w353:errorcluster)
            n112 = Unbundle By Name(w357) -> ("Device Name"=w356:T2, "Value"=w355:bool, "Index"=w354:i32)
            n113 = call "DCON Action Engine.vi"("Index\\Channel"=w354, "Action"=DCON_Action_Engine-States."Set DO Value", "error in (no error)"=w353, "DO Value"=w355, "Device Name"=w356, "IO In"=w361) -> ("error out"=w360:errorcluster)  [unwired: 2 in, 3 out]
          }
          frame Enabled {
          }
        }
        n114 = disable-structure shown="Enabled" {
          disable-tunnel: w337 -> [w349 _]
          disable-tunnel: w336 -> [w348 _]
          disable-tunnel: [w347 w351] -> w335
          disable-tunnel: w334 -> [w346 w351]
          frame Enabled {
            n115 = call <vilib>:"Add State to Queue with vData.vi"("queue in"=w349, "mode (back)"=enum16{"back", "front"}."back", "state in"="Set DO Value", "vData (\"\")"=w348, "error in"=w346) -> ("error out"=w347:errorcluster)  [unwired: 7 in, 3 out]
          }
          frame Disabled {
          }
        }
        n116 = call <vilib>:"Add State(s) to Queue__JKI_lib_State_Machine.vi"("State(s) in Front (\"\")"="Task: Completed" ("State(s) in Front (\"\")"), "State(s) in (\"\")"=w339) -> ("States Out"=w340:string)  [unwired: 13 in]
      }
      frame "API: Set AO Value" {
        n117 = Unbundle By Name(w375) -> ("TopLevel out"=w373:refnum<class "IO.lvclass">, "Current Task.Data"=w365:variant)
        n118 = disable-structure shown="Disabled" {
          disable-tunnel: w374 -> [w387 w388]
          disable-tunnel: w373 -> [w386 _]
          disable-tunnel: [w378 w388] -> w368
          disable-tunnel: w365 -> [w377 _]
          frame Disabled {
            n119 = Variant To Data(error in=w387, type=T23 {"Device Name"=enum."ICP1-DO", "Index"=0, "Value"=0.0} ("DO Value Input"), Variant=w377) -> (data=w383:T23, error out=w385:errorcluster)
            n120 = Unbundle By Name(w383) -> ("Value"=w379:dbl, "Device Name"=w382:T2, "Index"=w381:i32)
            n121 = call "DCON Action Engine.vi"("Index\\Channel"=w381, "AO Value"=w379, "Action"=DCON_Action_Engine-States."Set AO Value", "error in (no error)"=w385, "Device Name"=w382, "IO In"=w386) -> ("error out"=w378:errorcluster)  [unwired: 2 in, 3 out]
          }
          frame Enabled {
          }
        }
        n122 = call <vilib>:"Add State to Queue with vData.vi"("queue in"=w366, "mode (back)"=enum16{"back", "front"}."front", "state in"="Set AO Value", "vData (\"\")"=w365, "error in"=w368) -> ("error out"=w367:errorcluster)  [unwired: 7 in, 3 out]
        n123 = call <vilib>:"Add State(s) to Queue__JKI_lib_State_Machine.vi"("State(s) in Front (\"\")"="Task: Completed" ("State(s) in Front (\"\")"), "State(s) in (\"\")"=w370) -> ("States Out"=w371:string)  [unwired: 13 in]
      }
      frame "API: Purge PH" {
        n124 = Unbundle By Name(w406) -> ("Current Task.Data"=w400:variant, "TopLevel out"=w395:refnum<class "IO.lvclass">)
        n125 = Variant To Data(error in=w396, type=T24 {"ICP1-DO Channel Name"=enum."None", "Duration (s)"=3.0} ("Purge PH API Data"), Variant=w400) -> (data=w398:T24, error out=w392:errorcluster)
        n126 = Unbundle By Name(w398) -> ("Duration (s)"=w397:dbl, "ICP1-DO Channel Name"=w393:T25)
        n127 = call-dynamic "Get Ordered Channels_Digital_Status_IO.vi"("error in (no error)"=w392, "IO in"=w395) -> ("error out"=w391:errorcluster, "IO out"=w389:refnum<class "IO.lvclass">, "Ordered ICP1-DO Channels"=w394:T25[])  [unwired: 5 in, 2 out]
        n128 = Search 1D Array(1D array=w394, element=w393) -> (index of element=w390:i32)  [unwired: 1 in]
        n129 = case shown="Default" w390 {
          selector: w390 -> [_ w409]
          tunnel: [w408 w429] -> w402
          tunnel: w401 -> [_ w426]
          tunnel: w397 -> [_ w424]
          tunnel: w391 -> [w408 w419]
          tunnel: w389 -> [_ w415]
          frame -1 {
          }
          frame Default {
            w410 = FALSE ("Value")
            w413 = TRUE ("Value")
            w411 = Device_Names."ICP1-DO" ("Device Name")
            w414 = Device_Names."ICP1-DO" ("Device Name")
            n130 = Bundle By Name(cluster=T22 {"Device Name"=enum."ICP1-DO", "Value"=FALSE, "Index"=0} ("DO Value Input"), "Device Name"=w414, "Value"=w413, "Index"=w409) -> (w421:T22)
            n131 = Multiply(x=w424, y=1000.0 ("x")) -> (x*y=w418:dbl)
            n132 = To Unsigned Long Integer(number=w418) -> (unsigned 32bit integer=w416:u32)
            n133 = disable-structure shown="Enabled" {
              disable-tunnel: [w447 w451] -> w428
              disable-tunnel: w426 -> [w446 w450]
              disable-tunnel: [w445 w450] -> w425
              disable-tunnel: w421 -> [w444 _]
              disable-tunnel: w419 -> [w443 w452]
              disable-tunnel: w415 -> [_ w457]
              disable-tunnel: w414 -> [_ w456]
              disable-tunnel: w413 -> [_ w455]
              disable-tunnel: w409 -> [_ w454]
              disable-tunnel: [_ w453] -> w412
              frame Disabled {
                n134 = call <vilib>:"Add State to Queue with vData.vi"("queue in"=w446, "mode (back)"=enum16{"back", "front"}."front", "state in"="Set DO Value", "vData (\"\")"=w444, "error in"=w443) -> ("queue out"=w445:refnum<queue>, "error out"=w447:errorcluster)  [unwired: 7 in, 2 out]
              }
              frame Enabled {
                n135 = call "DCON Action Engine.vi"("Index\\Channel"=w454, "Action"=DCON_Action_Engine-States."Set DO Value", "error in (no error)"=w452, "DO Value"=w455, "Device Name"=w456, "IO In"=w457) -> ("error out"=w451:errorcluster, "IO Out"=w453:refnum<class "IO.lvclass">)  [unwired: 2 in, 2 out]
              }
            }
            n136 = Bundle By Name(cluster=T22 {"Device Name"=enum."ICP1-DO", "Value"=FALSE, "Index"=0} ("DO Value Input"), "Device Name"=w411, "Value"=w410, "Index"=w409) -> (w420:T22)
            n137 = call <userlib>:"Wait (ms)__ogtk.vi"("error in (no error)"=w428, "milliseconds to wait"=w416) -> ("error out"=w427:errorcluster)  [unwired: 8 in, 1 out]
            n138 = disable-structure shown="Enabled" {
              disable-tunnel: [w433 w436] -> w429
              disable-tunnel: w427 -> [w432 w437]
              disable-tunnel: w425 -> [w431 _]
              disable-tunnel: w420 -> [w430 _]
              disable-tunnel: w412 -> [_ w441]
              disable-tunnel: w411 -> [_ w440]
              disable-tunnel: w410 -> [_ w439]
              disable-tunnel: w409 -> [_ w438]
              frame Disabled {
                n139 = call <vilib>:"Add State to Queue with vData.vi"("queue in"=w431, "mode (back)"=enum16{"back", "front"}."front", "state in"="Set DO Value", "vData (\"\")"=w430, "error in"=w432) -> ("error out"=w433:errorcluster)  [unwired: 7 in, 3 out]
              }
              frame Enabled {
                n140 = call "DCON Action Engine.vi"("Index\\Channel"=w438, "Action"=DCON_Action_Engine-States."Set DO Value", "error in (no error)"=w437, "DO Value"=w439, "Device Name"=w440, "IO In"=w441) -> ("error out"=w436:errorcluster)  [unwired: 2 in, 3 out]
              }
            }
          }
        }
        n141 = call <vilib>:"Add State(s) to Queue__JKI_lib_State_Machine.vi"("State(s) in Front (\"\")"="Task: Completed" ("State(s) in Front (\"\")"), "State(s) in (\"\")"=w403) -> ("States Out"=w404:string)  [unwired: 13 in]
      }
      frame "---------- Tasks ----------" {
      }
      frame "Task: Completed" {
        n142 = Unbundle By Name(w469) -> ("API Executed Event"=w467:refnum<user-event>, "Tasks"=w466:T16[], "Current Task. Return Value"=w463:variant)
        n143 = Empty Array?(array=w466) -> (empty?=w468:bool)
        n144 = case shown="False" w468 {
          tunnel: w467 -> [w478 _]
          tunnel: w466 -> [w479 _]
          tunnel: w464 -> [w476 w480]
          tunnel: [w475 w480] -> w465
          tunnel: w463 -> [w472 _]
          frame False {
            n145 = Index Array(array=w479) -> (element=w477:T16)  [unwired: 1 in]
            n146 = Bundle By Name(cluster=w477, "Task.Task State"=API_Task_State."Completed", "Return Value"=w472) -> (w474:T16)
            n147 = Generate User Event(user event=w478, event data cluster=w474, error in=w476) -> (error out=w475:errorcluster)  [unwired: 1 in, 1 out]
          }
          frame True {
          }
        }
      }
      frame "Task: Check Timeout" {
        n148 = Unbundle By Name(w488) -> ("API Executed Event"=w486:refnum<user-event>, "Task Start ms"=w481:u32, "Tasks"=w483:T16[])
        n149 = Index Array(array=w483) -> (element=w482:T16)  [unwired: 1 in]
        n150 = Empty Array?(array=w483) -> (empty?=w487:bool)
        n151 = case shown="False" w487 {
          tunnel: w486 -> [w492 _]
          tunnel: w484 -> [w498 w507]
          tunnel: [w493 w507] -> w485
          tunnel: w482 -> [w497 _]
          tunnel: w481 -> [w501 _]
          frame False {
            n152 = Unbundle By Name(w497) -> ("Task.Timeout (ms)"=w499:u32)
            n153 = Tick Count (ms)() -> (millisecond timer value=w491:u32)
            n154 = Subtract(x=w491, y=w501) -> (x-y=w500:u32)
            n155 = Bundle By Name(cluster=w497, "Task.Task State"=API_Task_State."Errored") -> (w495:T16)
            n156 = Greater Or Equal?(x=w500, y=w499) -> (x >= y?=w494:bool)
            n157 = case shown="False" w494 {
              tunnel: w498 -> [w502 w506]
              tunnel: w495 -> [_ w504]
              tunnel: [w502 w505] -> w493
              tunnel: w492 -> [_ w503]
              frame False {
              }
              frame True {
                n158 = Generate User Event(user event=w503, event data cluster=w504, error in=w506) -> (error out=w505:errorcluster)  [unwired: 1 in, 1 out]
              }
            }
          }
          frame True {
          }
        }
      }
      frame "Task: Check Pending" {
        n159 = Unbundle By Name(w508) -> ("API Executed Event"=w517:refnum<user-event>, "Task Start ms"=w514:u32, "Tasks"=w513:T16[])
        n160 = Empty Array?(array=w513) -> (empty?=w518:bool)
        n161 = case shown="False" w518 {
          tunnel: w517 -> [_ _]
          tunnel: w515 -> [w528 w537]
          tunnel: [w526 w537] -> w516
          tunnel: w514 -> [_ _]
          tunnel: w513 -> [w535 _]
          tunnel: [w525 _] -> w510
          tunnel: w508 -> [w524 w536]
          tunnel: [w522 w536] -> w509
          frame False {
            n162 = Index Array(array=w535) -> (element=w530:T16)  [unwired: 1 in]
            n163 = Unbundle By Name(w530) -> ("Command"=w529:variant)
            n164 = Tick Count (ms)() -> (millisecond timer value=w523:u32)
            n165 = Variant To Data(error in=w528, type=T18 {"Command"=enum."Set DO Value", "Arguments"="", "Data"=variant} ("API Command Cluster"), Variant=w529) -> (data=w520:T18, error out=w527:errorcluster)
            n166 = Unbundle By Name(w520) -> ("Command"=w532:T19, "Arguments"=w531:string)
            n167 = Bundle By Name(cluster=w524, "TO"=100, "Task Start ms"=w523, "Current Task"=w520) -> (w522:T32)
            n168 = Format Into String(format string="API: %s>>%s", error in=w527, w532, w531) -> (resulting string=w525:string, error out=w526:errorcluster)  [unwired: 1 in]
          }
          frame True {
          }
        }
        n169 = call <vilib>:"Add State(s) to Queue__JKI_lib_State_Machine.vi"("State(s) in Front (\"\")"=w510, "State(s) in (\"\")"=w511) -> ("States Out"=w512:string)  [unwired: 13 in]
      }
      frame "Task: Remove on Error" {
        n170 = Unbundle By Name(w543) -> ("API Return Event"=w545:refnum<user-event>, "Tasks"=w544:T16[])
        n171 = for {
          tunnel: w545 -> [w555]
          tunnel: w544 -> [w554] mode=indexing
          shift-right: [w549] -> w542
          shift-left: w541 -> [w550]
          n172 = Get Date/Time In Seconds() -> (seconds since 1Jan1904=w551:timestamp)
          n173 = Bundle By Name(cluster=w554, "Task.Task State"=API_Task_State."Errored", "Task.Time Stamp"=w551) -> (w553:T16)
          n174 = Generate User Event(user event=w555, event data cluster=w553, error in=w550) -> (error out=w549:errorcluster)  [unwired: 1 in, 1 out]
        }
        n175 = Bundle By Name(cluster=w543, "TO"=-1, "Tasks"=T16[] []) -> (w540:T32)
        n176 = call <vilib>:"Add State(s) to Queue__JKI_lib_State_Machine.vi"("State(s) in (\"\")"=w546) -> ("States Out"=w547:string)  [unwired: 14 in]
      }
      frame "-----------Init----------------" {
      }
      frame "Init: DCON Open" {
        n177 = Unbundle By Name(w569) -> ("Methods:Accessors:Digilens Config.IO Config.DAQDevices"=w565:T7[], "TopLevel out"=w568:refnum<class "IO.lvclass">)
        n178 = call "DCON Action Engine.vi"("Action"=DCON_Action_Engine-States."Open", "DAQDevices"=w565, "error in (no error)"=w567, "IO In"=w568) -> ("error out"=w564:errorcluster)  [unwired: 4 in, 3 out]
        n179 = Unbundle By Name(w564) -> ("status"=w561:bool)
        n180 = case shown="False" w561 {
          tunnel: w563 -> [w574 _]
          tunnel: [w572 _] -> _
          frame False {
            n181 = call <vilib>:"Add State to Queue with vData.vi"("queue in"=w574, "state in"="UpdateSettings>>Open", "vData (\"\")"=TRUE) -> ("error out"=w572:errorcluster)  [unwired: 9 in, 3 out]
          }
          frame True {
          }
        }
        n182 = Not(x=w561) -> (.not. x?=w560:bool)
        n183 = Bundle By Name(cluster=w569, "DCONOpen"=w560) -> (w562:T32)
      }
      frame "Init: Set ICP2-DI Channels" {
        n184 = Unbundle By Name(w581) -> ("TopLevel out"=w577:refnum<class "IO.lvclass">, "Methods:Accessors:Digilens Config.IO Config.DI Channels"=w580:T8[], "DCONOpen"=w576:bool)
        n185 = case shown="True" w576 {
          tunnel: w580 -> [_ w602]
          tunnel: [w584 w598] -> w579
          tunnel: w578 -> [w584 w594]
          tunnel: w577 -> [_ w593]
          frame False {
          }
          frame True {
            n186 = call "DCON Action Engine.vi"("Action"=DCON_Action_Engine-States."Get Data", "error in (no error)"=w594, "Device Name"=Device_Names."ICP2-DI" ("Device Names"), "IO In"=w593) -> ("error out"=w589:errorcluster, "Status Out"=w591:T36, "IO Out"=w592:refnum<class "IO.lvclass">)  [unwired: 4 in, 1 out]
            n187 = Unbundle By Name(w591) -> ("DeviceName"=w585:string, "Number of Channels"=w590:i32)
            n188 = for {
              tunnel: w602 -> [w618] mode=indexing
              tunnel: [w617] -> w601 mode=indexing if=w614
              tunnel: w585 -> [w613]
              n189 = Unbundle By Name(w618) -> ("Device Name"=w615:string, "Channel No"=w619:string)
              n190 = Equal?(x=w615, y=w613) -> (x = y?=w614:bool)
              n191 = Decimal String To Number(string=w619) -> (number=w616:i32)  [unwired: 2 in, 1 out]
              n192 = Bundle(w616, "Channel"=w618) -> (w617:cluster{i32, "Channel":T8})  [unwired: 1 in]
            }
            n193 = Sort 1D Array(array=w601) -> (sorted array=w600:cluster{i32, "Channel":T8}[])
            n194 = Initialize Array(ICP2-DI_Channel_Names."None" ("DI Channels"), w590) -> (w596:T26[])
            n195 = for {
              tunnel: w600 -> [w612] mode=indexing
              tunnel: ICP2-DI_Channel_Names."None" ("DI Channels") -> [w610]
              shift-right: [w607] -> w587
              shift-left: w596 -> [w608]
              shift-right: [w605] -> w588
              shift-left: w589 -> [w606]
              n196 = Unbundle(w612) -> (w603:i32, "Channel"=w611:T8)
              n197 = Unbundle By Name(w611) -> ("Channel Name"=w609:string)
              n198 = Scan From String(input string=w609, error in=w606, default 1=w610) -> (error out=w605:errorcluster, output 1=w604:T26)  [unwired: 2 in, 2 out]
              n199 = Insert Into Array(array=w608, index=w603, new element=w604) -> (w607:T26[])
            }
            n200 = call-dynamic "Set Ordered ICP2-DI Channels_Status_IO.vi"("error in (no error)"=w588, "Ordered ICP2-DI Channels"=w587, "IO in"=w592) -> ("error out"=w598:errorcluster)  [unwired: 7 in, 1 out]
          }
        }
      }
      frame "Init: Set ICP2-DO Channels" {
        n201 = Unbundle By Name(w625) -> ("TopLevel out"=w621:refnum<class "IO.lvclass">, "Methods:Accessors:Digilens Config.IO Config.DO Channels"=w624:T8[], "DCONOpen"=w620:bool)
        n202 = case shown="True" w620 {
          tunnel: w624 -> [_ w646]
          tunnel: [w628 w643] -> w623
          tunnel: w622 -> [w628 w640]
          tunnel: w621 -> [_ w639]
          frame False {
          }
          frame True {
            n203 = call "DCON Action Engine.vi"("Action"=DCON_Action_Engine-States."Get Data", "error in (no error)"=w640, "Device Name"=Device_Names."ICP2-DO" ("Device Names"), "IO In"=w639) -> ("error out"=w631:errorcluster, "Status Out"=w638:T36, "IO Out"=w632:refnum<class "IO.lvclass">)  [unwired: 4 in, 1 out]
            n204 = Unbundle By Name(w638) -> ("DeviceName"=w629:string, "Number of Channels"=w637:i32)
            n205 = for {
              tunnel: w646 -> [w662] mode=indexing
              tunnel: [w661] -> w645 mode=indexing if=w657
              tunnel: w629 -> [w658]
              n206 = Unbundle By Name(w662) -> ("Device Name"=w659:string, "Channel No"=w663:string)
              n207 = Equal?(x=w659, y=w658) -> (x = y?=w657:bool)
              n208 = Decimal String To Number(string=w663) -> (number=w660:i32)  [unwired: 2 in, 1 out]
              n209 = Bundle(w660, "Channel"=w662) -> (w661:cluster{i32, "Channel":T8})  [unwired: 1 in]
            }
            n210 = Sort 1D Array(array=w645) -> (sorted array=w644:cluster{i32, "Channel":T8}[])
            n211 = Initialize Array(ICP2-DO_Channel_Names."None" ("DO Channel Names"), w637) -> (w642:T27[])
            n212 = for {
              tunnel: w644 -> [w656] mode=indexing
              tunnel: ICP2-DO_Channel_Names."None" ("DO Channel Names") -> [w654]
              shift-right: [w651] -> w635
              shift-left: w642 -> [w652]
              shift-right: [w649] -> w636
              shift-left: w631 -> [w650]
              n213 = Unbundle(w656) -> (w647:i32, "Channel"=w655:T8)
              n214 = Unbundle By Name(w655) -> ("Channel Name"=w653:string)
              n215 = Scan From String(input string=w653, error in=w650, default 1=w654) -> (error out=w649:errorcluster, output 1=w648:T27)  [unwired: 2 in, 2 out]
              n216 = Insert Into Array(array=w652, index=w647, new element=w648) -> (w651:T27[])
            }
            n217 = call-dynamic "Set Ordered ICP2-DO Channels_Status_IO.vi"("error in (no error)"=w636, "Ordered ICP2-DO Channels"=w635, "IO in"=w632) -> ("error out"=w643:errorcluster)  [unwired: 7 in, 1 out]
          }
        }
      }
      frame "Init: Set ICP1-DO Channels" {
        n218 = Unbundle By Name(w669) -> ("TopLevel out"=w665:refnum<class "IO.lvclass">, "Methods:Accessors:Digilens Config.IO Config.DO Channels"=w668:T8[], "DCONOpen"=w664:bool)
        n219 = case shown="True" w664 {
          tunnel: w668 -> [_ w690]
          tunnel: [w672 w687] -> w667
          tunnel: w666 -> [w672 w684]
          tunnel: w665 -> [_ w683]
          frame False {
          }
          frame True {
            n220 = call "DCON Action Engine.vi"("Action"=DCON_Action_Engine-States."Get Data", "error in (no error)"=w684, "Device Name"=Device_Names."ICP1-DO" ("Device Names"), "IO In"=w683) -> ("error out"=w675:errorcluster, "Status Out"=w682:T36, "IO Out"=w676:refnum<class "IO.lvclass">)  [unwired: 4 in, 1 out]
            n221 = Unbundle By Name(w682) -> ("DeviceName"=w673:string, "Number of Channels"=w681:i32)
            n222 = for {
              tunnel: w690 -> [w706] mode=indexing
              tunnel: [w705] -> w689 mode=indexing if=w701
              tunnel: w673 -> [w702]
              n223 = Unbundle By Name(w706) -> ("Device Name"=w703:string, "Channel No"=w707:string)
              n224 = Equal?(x=w703, y=w702) -> (x = y?=w701:bool)
              n225 = Decimal String To Number(string=w707) -> (number=w704:i32)  [unwired: 2 in, 1 out]
              n226 = Bundle(w704, "Channel"=w706) -> (w705:cluster{i32, "Channel":T8})  [unwired: 1 in]
            }
            n227 = Sort 1D Array(array=w689) -> (sorted array=w688:cluster{i32, "Channel":T8}[])
            n228 = Initialize Array(ICP1-D0_Channel_Names."None" ("ICP1-DO Channel Names"), w681) -> (w686:T25[])
            n229 = for {
              tunnel: w688 -> [w700] mode=indexing
              tunnel: ICP1-D0_Channel_Names."None" ("ICP1-DO Channel Names") -> [w698]
              shift-right: [w695] -> w679
              shift-left: w686 -> [w696]
              shift-right: [w693] -> w680
              shift-left: w675 -> [w694]
              n230 = Unbundle(w700) -> (w691:i32, "Channel"=w699:T8)
              n231 = Unbundle By Name(w699) -> ("Channel Name"=w697:string)
              n232 = Scan From String(input string=w697, error in=w694, default 1=w698) -> (error out=w693:errorcluster, output 1=w692:T25)  [unwired: 2 in, 2 out]
              n233 = Insert Into Array(array=w696, index=w691, new element=w692) -> (w695:T25[])
            }
            n234 = call-dynamic "Set Ordered ICP1-DO Channels_Status_IO.vi"("error in (no error)"=w680, "Ordered ICP1-DO Channels"=w679, "IO in"=w676) -> ("error out"=w687:errorcluster)  [unwired: 7 in, 1 out]
          }
        }
      }
      frame "Init: Set ICP1-AI Channels" {
        n235 = Unbundle By Name(w713) -> ("TopLevel out"=w709:refnum<class "IO.lvclass">, "Methods:Accessors:Digilens Config.IO Config.AI Channels"=w712:T8[], "DCONOpen"=w708:bool)
        n236 = case shown="True" w708 {
          tunnel: w712 -> [_ w734]
          tunnel: [w716 w731] -> w711
          tunnel: w710 -> [w716 w728]
          tunnel: w709 -> [_ w727]
          frame False {
          }
          frame True {
            n237 = call "DCON Action Engine.vi"("Action"=DCON_Action_Engine-States."Get Data", "error in (no error)"=w728, "Device Name"=Device_Names."ICP1-DO" ("Device Names"), "IO In"=w727) -> ("error out"=w719:errorcluster, "Status Out"=w726:T36, "IO Out"=w720:refnum<class "IO.lvclass">)  [unwired: 4 in, 1 out]
            n238 = Unbundle By Name(w726) -> ("DeviceName"=w717:string, "Number of Channels"=w725:i32)
            n239 = for {
              tunnel: w734 -> [w750] mode=indexing
              tunnel: [w749] -> w733 mode=indexing if=w745
              tunnel: w717 -> [w746]
              n240 = Unbundle By Name(w750) -> ("Device Name"=w747:string, "Channel No"=w751:string)
              n241 = Equal?(x=w747, y=w746) -> (x = y?=w745:bool)
              n242 = Decimal String To Number(string=w751) -> (number=w748:i32)  [unwired: 2 in, 1 out]
              n243 = Bundle(w748, "Channel"=w750) -> (w749:cluster{i32, "Channel":T8})  [unwired: 1 in]
            }
            n244 = Sort 1D Array(array=w733) -> (sorted array=w732:cluster{i32, "Channel":T8}[])
            n245 = Initialize Array(ICP1-AI_Channel_Names."None" ("ICP1-AI Channel Names"), w725) -> (w730:T28[])
            n246 = for {
              tunnel: w732 -> [w744] mode=indexing
              tunnel: ICP1-AI_Channel_Names."None" ("ICP1-AI Channel Names") -> [w742]
              shift-right: [w739] -> w723
              shift-left: w730 -> [w740]
              shift-right: [w737] -> w724
              shift-left: w719 -> [w738]
              n247 = Unbundle(w744) -> (w735:i32, "Channel"=w743:T8)
              n248 = Unbundle By Name(w743) -> ("Channel Name"=w741:string)
              n249 = Scan From String(input string=w741, error in=w738, default 1=w742) -> (error out=w737:errorcluster, output 1=w736:T28)  [unwired: 2 in, 2 out]
              n250 = Insert Into Array(array=w740, index=w735, new element=w736) -> (w739:T28[])
            }
            n251 = call-dynamic "Set Ordered ICP1-AI Channels_Status_IO.vi"("error in (no error)"=w724, "Ordered ICP1-AI Channels"=w723, "IO in"=w720) -> ("error out"=w731:errorcluster)  [unwired: 7 in, 1 out]
          }
        }
      }
      frame "Init: Set ICP1-AO Channels" {
        n252 = Unbundle By Name(w757) -> ("TopLevel out"=w753:refnum<class "IO.lvclass">, "Methods:Accessors:Digilens Config.IO Config.AO Channels"=w756:T8[], "DCONOpen"=w752:bool)
        n253 = case shown="True" w752 {
          tunnel: w756 -> [_ w778]
          tunnel: [w760 w775] -> w755
          tunnel: w754 -> [w760 w772]
          tunnel: w753 -> [_ w771]
          frame False {
          }
          frame True {
            n254 = call "DCON Action Engine.vi"("Action"=DCON_Action_Engine-States."Get Data", "error in (no error)"=w772, "Device Name"=Device_Names."ICP1-AO" ("Device Names"), "IO In"=w771) -> ("error out"=w763:errorcluster, "Status Out"=w770:T36, "IO Out"=w764:refnum<class "IO.lvclass">)  [unwired: 4 in, 1 out]
            n255 = Unbundle By Name(w770) -> ("DeviceName"=w761:string, "Number of Channels"=w769:i32)
            n256 = for {
              tunnel: w778 -> [w794] mode=indexing
              tunnel: [w793] -> w777 mode=indexing if=w789
              tunnel: w761 -> [w790]
              n257 = Unbundle By Name(w794) -> ("Device Name"=w791:string, "Channel No"=w795:string)
              n258 = Equal?(x=w791, y=w790) -> (x = y?=w789:bool)
              n259 = Decimal String To Number(string=w795) -> (number=w792:i32)  [unwired: 2 in, 1 out]
              n260 = Bundle(w792, "Channel"=w794) -> (w793:cluster{i32, "Channel":T8})  [unwired: 1 in]
            }
            n261 = Sort 1D Array(array=w777) -> (sorted array=w776:cluster{i32, "Channel":T8}[])
            n262 = Initialize Array(ICP1-AO_Channel_Names."None" ("ICP1-AO Channel Names"), w769) -> (w774:T29[])
            n263 = for {
              tunnel: w776 -> [w788] mode=indexing
              tunnel: ICP1-AO_Channel_Names."None" ("ICP1-AO Channel Names") -> [w786]
              shift-right: [w783] -> w767
              shift-left: w774 -> [w784]
              shift-right: [w781] -> w768
              shift-left: w763 -> [w782]
              n264 = Unbundle(w788) -> (w779:i32, "Channel"=w787:T8)
              n265 = Unbundle By Name(w787) -> ("Channel Name"=w785:string)
              n266 = Scan From String(input string=w785, error in=w782, default 1=w786) -> (error out=w781:errorcluster, output 1=w780:T29)  [unwired: 2 in, 2 out]
              n267 = Insert Into Array(array=w784, index=w779, new element=w780) -> (w783:T29[])
            }
            n268 = call-dynamic "Set Ordered ICP1-AO Channels_Status_IO.vi"("error in (no error)"=w768, "Ordered ICP1-AO Channels"=w767, "IO in"=w764) -> ("error out"=w775:errorcluster)  [unwired: 7 in, 1 out]
          }
        }
      }
      frame "Init: Set ICP2-AO Channels" {
        n269 = Unbundle By Name(w801) -> ("TopLevel out"=w797:refnum<class "IO.lvclass">, "Methods:Accessors:Digilens Config.IO Config.AO Channels"=w800:T8[], "DCONOpen"=w796:bool)
        n270 = case shown="True" w796 {
          tunnel: w800 -> [_ w822]
          tunnel: [w804 w819] -> w799
          tunnel: w798 -> [w804 w816]
          tunnel: w797 -> [_ w815]
          frame False {
          }
          frame True {
            n271 = call "DCON Action Engine.vi"("Action"=DCON_Action_Engine-States."Get Data", "error in (no error)"=w816, "Device Name"=Device_Names."ICP2-AO" ("Device Names"), "IO In"=w815) -> ("error out"=w807:errorcluster, "Status Out"=w814:T36, "IO Out"=w808:refnum<class "IO.lvclass">)  [unwired: 4 in, 1 out]
            n272 = Unbundle By Name(w814) -> ("DeviceName"=w805:string, "Number of Channels"=w813:i32)
            n273 = for {
              tunnel: w822 -> [w838] mode=indexing
              tunnel: [w837] -> w821 mode=indexing if=w833
              tunnel: w805 -> [w834]
              n274 = Unbundle By Name(w838) -> ("Device Name"=w835:string, "Channel No"=w839:string)
              n275 = Equal?(x=w835, y=w834) -> (x = y?=w833:bool)
              n276 = Decimal String To Number(string=w839) -> (number=w836:i32)  [unwired: 2 in, 1 out]
              n277 = Bundle(w836, "Channel"=w838) -> (w837:cluster{i32, "Channel":T8})  [unwired: 1 in]
            }
            n278 = Sort 1D Array(array=w821) -> (sorted array=w820:cluster{i32, "Channel":T8}[])
            n279 = Initialize Array(ICP2-AO_Channel_Names."None" ("ICP2-AO Channel Names"), w813) -> (w818:T30[])
            n280 = for {
              tunnel: w820 -> [w832] mode=indexing
              tunnel: ICP2-AO_Channel_Names."None" ("ICP2-AO Channel Names") -> [w830]
              shift-right: [w827] -> w811
              shift-left: w818 -> [w828]
              shift-right: [w825] -> w812
              shift-left: w807 -> [w826]
              n281 = Unbundle(w832) -> (w823:i32, "Channel"=w831:T8)
              n282 = Unbundle By Name(w831) -> ("Channel Name"=w829:string)
              n283 = Scan From String(input string=w829, error in=w826, default 1=w830) -> (error out=w825:errorcluster, output 1=w824:T30)  [unwired: 2 in, 2 out]
              n284 = Insert Into Array(array=w828, index=w823, new element=w824) -> (w827:T30[])
            }
            n285 = call-dynamic "Set Ordered ICP2-AO Channels_Status_IO.vi"("error in (no error)"=w812, "Ordered ICP2-AO Channels"=w811, "IO in"=w808) -> ("error out"=w819:errorcluster)  [unwired: 7 in, 1 out]
          }
        }
      }
    }
  }
  n286 = Bundle By Name(cluster=T15 {"IOLoopEvents"=refnum, "Open"=FALSE, "Digilens Config"={"Motion Controller"={"Motor IP Addresss"="", "Current Position"=0, "Pulse_Per_mm"=0, "PrePrint"=[], "Load Position_mm"=0, "Laminate Position_mm"=0}, "IO Config"={"DAQDevices"=[], "DI Channels"=[], "DO Channels"=[], "Material Names"=[], "AI Channels"=[], "AO Channels"=[]}, "PrinterConfiguration"={"IPAddress"="", "Move Stage on RTP Command?"=FALSE, "Stage Move Position"="", "PH1-Prime Path"=path "", "PH2-Prime Path"=path "", "PH3-Prime Path"=path "", "PH4-Prime Path"=path "", "PH5-Prime Path"=path "", "PH6-Prime Path"=path "", "PrintScriptsFolder"=path "", "PurgeScriptsFolder"=path "", "StageScriptsFolder"=path "", "PH1-HeatOn Path"=path "", "PH2-HeatOn Path"=path "", "PH3-HeatOn Path"=path "", "PH4-HeatOn Path"=path "", "PH5-HeatOn Path"=path "", "PH6-HeatOn Path"=path "", "PH1-HeatOff Path"=path "", "PH2-HeatOff Path"=path "", "PH3-HeatOff Path"=path "", "PH4-HeatOff Path"=path "", "PH5-HeatOff Path"=path "", "PH6-HeatOff Path"=path ""}, "DAQ Settings"={"Simulate DAQ"=FALSE, "DI Settings"=[], "AI Settings"=[], "Relay IONames"=[], "AO IONames"=[], "AO NChan SingleTask"=FALSE}}}, "IOLoopEvents"=w5) -> (w9:T15)
  n287 = while {
    tunnel: w11 -> [w847]
    shift-right: [w851] -> w7
    shift-left: w12 -> [w853]
    shift-right: [w848] -> w4
    shift-left: w9 -> [w849]
    shift-right: [w840] -> _
    shift-left: "IO in" -> [w841]
    tunnel: w8 -> [_]
    stop <- w854 stop-if-true
    n288 = call <vilib>:"Get Next Queued State with vData.vi"("queue in"=w847, "error in (no error)"=w853) -> ("vData out"=w850:variant, "queue out"=w846:refnum<queue>, "Next State"=w845:string, "queued msg"=w842:string, "error out"=w852:errorcluster)  [unwired: 7 in, 2 out]
    n289 = call <vilib>:"Parse State Queue__JKI_lib_State_Machine.vi"("State Queue"=w845) -> ("Current State"=w844:string, "Arguments"=w843:string)  [unwired: 12 in, 1 out]
    n290 = case shown="\"Set DO Value\"" w844 {
      tunnel: [_ _ _ _ _ _ _ _ _ TRUE] -> w854
      tunnel: w852 -> [w857 w862 w877 w884 w899 w906 w962 w969 w988 w1002]
      tunnel: [w857 w860 w876 w885 w899 w905 errorcluster {"status"=FALSE, "code"=0, "source"=""} ("error out") w968 w997 w1002] -> w851
      tunnel: w850 -> [_ w863 w878 w886 _ _ _ w970 _ _]
      tunnel: w849 -> [w856 w861 w871 w894 w898 w904 w961 w967 w992 w1001]
      tunnel: [w856 w861 w871 w894 w897 w903 w961 w966 w996 w1001] -> w848
      tunnel: w846 -> [_ _ _ _ _ w900 _ _ w999 _]
      tunnel: w843 -> [_ _ _ _ _ _ _ _ _ _]
      tunnel: w842 -> [_ _ _ _ _ _ _ w965 _ _]
      tunnel: w841 -> [w855 w858 w872 w883 w895 w902 w960 w964 w990 w1000]
      tunnel: [w855 w859 w875 w882 w895 w901 w960 w964 w991 w1000] -> w840
      frame Default {
      }
      frame "Set DO Value" {
        n291 = Variant To Data(error in=w862, type=T22 {"Device Name"=enum."ICP1-DO", "Value"=FALSE, "Index"=0} ("DO Value Input"), Variant=w863) -> (data=w868:T22, error out=w864:errorcluster)
        n292 = Unbundle By Name(w868) -> ("Device Name"=w867:T2, "Value"=w866:bool, "Index"=w865:i32)
        n293 = call "DCON Action Engine.vi"("Index\\Channel"=w865, "Action"=DCON_Action_Engine-States."Set DO Value", "error in (no error)"=w864, "DO Value"=w866, "Device Name"=w867, "IO In"=w858) -> ("error out"=w860:errorcluster, "IO Out"=w859:refnum<class "IO.lvclass">)  [unwired: 2 in, 2 out]
      }
      frame "ReadBack" {
        n294 = Variant To Data(error in=w877, type=T1 {"Device Name"=enum."ICP2-DI", "Action"=enum."Get AI Status"} ("ReadbackQuery"), Variant=w878) -> (data=w881:T1, error out=w879:errorcluster)
        n295 = Unbundle By Name(w881) -> ("Device Name"=w880:T2, "Action"=w873:T3)
        n296 = call "DCON Action Engine.vi"("Action"=w873, "error in (no error)"=w879, "Device Name"=w880, "IO In"=w872) -> ("error out"=w876:errorcluster, "IO Out"=w875:refnum<class "IO.lvclass">)  [unwired: 4 in, 2 out]
      }
      frame "Set AO Value" {
        n297 = Variant To Data(error in=w884, type=T23 {"Device Name"=enum."ICP1-DO", "Index"=0, "Value"=0.0} ("DO Value Input"), Variant=w886) -> (data=w891:T23, error out=w893:errorcluster)
        n298 = Unbundle By Name(w891) -> ("Value"=w887:dbl, "Device Name"=w890:T2, "Index"=w889:i32)
        n299 = call "DCON Action Engine.vi"("Index\\Channel"=w889, "AO Value"=w887, "Action"=DCON_Action_Engine-States."Set AO Value", "error in (no error)"=w893, "Device Name"=w890, "IO In"=w883) -> ("error out"=w885:errorcluster, "IO Out"=w882:refnum<class "IO.lvclass">)  [unwired: 2 in, 2 out]
      }
      frame "Initialize" {
        n300 = Bundle By Name(cluster=w898, "Open"=FALSE) -> (w897:T15)
      }
      frame "", "EventHandler", "Idle" {
        n301 = event shown="[0] Timeout" {
          selector: _ -> [_]
          dyn-events: _ -> [_]
          timeout: 200 -> [_]
          tunnel: w904 -> [w914]
          tunnel: w906 -> [w912]
          tunnel: [w911] -> w905
          tunnel: [w915] -> w903
          tunnel: w902 -> [w910]
          tunnel: [w909] -> w901
          tunnel: w900 -> [w908]
          event Timeout {
            n302 = event-data() -> ()  [unwired: 1 in, 3 out]
            n303 = Unbundle By Name(w914) -> ("Open"=w913:bool)
            n304 = case shown="False" w913 {
              tunnel: w914 -> [w918 w921]
              tunnel: [w918 w921] -> w915
              tunnel: w912 -> [w917 w923]
              tunnel: [w917 w922] -> w911
              tunnel: w910 -> [w916 w924]
              tunnel: [w916 w920] -> w909
              tunnel: w908 -> [_ w919]
              frame False {
              }
              frame True {
                n305 = disable-structure shown="Enabled" {
                  disable-tunnel: w924 -> [w934 w949]
                  disable-tunnel: w923 -> [w933 w953]
                  disable-tunnel: [w932 w950] -> w922
                  disable-tunnel: w921 -> [w931 _]
                  disable-tunnel: [w926 w949] -> w920
                  disable-tunnel: w919 -> [_ w952]
                  frame Disabled {
                    w925 = T3[] [enum."Get AI Status", enum."Get AO Status", enum."Get AO Status"] items=["Open", "Close", "Set DO Value", "Get Digital Status", "Get Data", "Get AI Status", "Set AO Value", "Get AO Status"]
                    w928 = T2[] [enum."ICP1-AI", enum."ICP1-AO", enum."ICP2-AO"] items=["ICP1-DO", "ICP2-DI", "ICP2-DO", "ICP1-AI", "ICP1-AO", "ICP2-AO"]
                    w930 = T2[] [enum."ICP2-DO", enum."ICP2-DI"] items=["ICP1-DO", "ICP2-DI", "ICP2-DO", "ICP1-AI", "ICP1-AO", "ICP2-AO"]
                    n306 = Unbundle By Name(w931) -> ("Digilens Config.IO Config.DAQDevices"=w929:T7[])
                    n307 = for {
                      tunnel: w929 -> [w945]
                      shift-right: [w946] -> w932
                      shift-left: w933 -> [w947]
                      tunnel: w930 -> [w943] mode=indexing
                      shift-right: [w942] -> w927
                      shift-left: w934 -> [w948]
                      n308 = call "DCON Action Engine.vi"("Action"=DCON_Action_Engine-States."Get Digital Status", "DAQDevices"=w945, "error in (no error)"=w947, "Device Name"=w943, "IO In"=w948) -> ("error out"=w946:errorcluster, "IO Out"=w942:refnum<class "IO.lvclass">)  [unwired: 3 in, 2 out]
                    }
                    n309 = for {
                      tunnel: w929 -> [w938]
                      shift-right: [w939] -> _
                      shift-left: _ -> [w940]
                      tunnel: w928 -> [w937] mode=indexing
                      shift-right: [w936] -> w926
                      shift-left: w927 -> [w941]
                      tunnel: w925 -> [w935] mode=indexing
                      n310 = call "DCON Action Engine.vi"("Action"=w935, "DAQDevices"=w938, "error in (no error)"=w940, "Device Name"=w937, "IO In"=w941) -> ("error out"=w939:errorcluster, "IO Out"=w936:refnum<class "IO.lvclass">)  [unwired: 3 in, 2 out]
                    }
                  }
                  frame Enabled {
                    n311 = for {
                      tunnel: w953 -> [w957]
                      tunnel: w952 -> [w958]
                      tunnel: T1[] [{"Device Name"=enum."ICP2-DO", "Action"=enum."Get Digital Status"}, {"Device Name"=enum."ICP2-DI", "Action"=enum."Get Digital Status"}, {"Device Name"=enum."ICP1-AI", "Action"=enum."Get AI Status"}] -> [w956] mode=indexing
                      tunnel: [w954] -> w950
                      n312 = call <vilib>:"Add State to Queue with vData.vi"("queue in"=w958, "mode (back)"=enum16{"back", "front"}."back", "state in"="ReadBack", "vData (\"\")"=w956, "error in"=w957) -> ("error out"=w954:errorcluster)  [unwired: 7 in, 3 out]
                    }
                  }
                }
              }
            }
          }
        }
      }
      frame "Error Handler" {
        n313 = call <vilib>:"General Error Handler.vi"("error in (no error)"=w962) -> ()  [unwired: 10 in, 5 out]
      }
      frame "UpdateSettings" {
        n314 = case shown="\"Open\"" w965 {
          tunnel: w970 -> [_ w976 w983]
          tunnel: w969 -> [w972 w977 w984]
          tunnel: [w972 w978 w985] -> w968
          tunnel: w967 -> [w971 w979 w986]
          tunnel: [w971 w974 w982] -> w966
          frame "False", Default {
          }
          frame "Configuration" {
            n315 = Variant To Data(error in=w977, type=T4 {"Motion Controller"={"Motor IP Addresss"="", "Current Position"=0, "Pulse_Per_mm"=0, "PrePrint"=[], "Load Position_mm"=0, "Laminate Position_mm"=0}, "IO Config"={"DAQDevices"=[], "DI Channels"=[], "DO Channels"=[], "Material Names"=[], "AI Channels"=[], "AO Channels"=[]}, "PrinterConfiguration"={"IPAddress"="", "Move Stage on RTP Command?"=FALSE, "Stage Move Position"="", "PH1-Prime Path"=path "", "PH2-Prime Path"=path "", "PH3-Prime Path"=path "", "PH4-Prime Path"=path "", "PH5-Prime Path"=path "", "PH6-Prime Path"=path "", "PrintScriptsFolder"=path "", "PurgeScriptsFolder"=path "", "StageScriptsFolder"=path "", "PH1-HeatOn Path"=path "", "PH2-HeatOn Path"=path "", "PH3-HeatOn Path"=path "", "PH4-HeatOn Path"=path "", "PH5-HeatOn Path"=path "", "PH6-HeatOn Path"=path "", "PH1-HeatOff Path"=path "", "PH2-HeatOff Path"=path "", "PH3-HeatOff Path"=path "", "PH4-HeatOff Path"=path "", "PH5-HeatOff Path"=path "", "PH6-HeatOff Path"=path ""}, "DAQ Settings"={"Simulate DAQ"=FALSE, "DI Settings"=[], "AI Settings"=[], "Relay IONames"=[], "AO IONames"=[], "AO NChan SingleTask"=FALSE}} ("Digilens Config"), Variant=w976) -> (data=w973:T4, error out=w978:errorcluster)
            n316 = Bundle By Name(cluster=w979, "Digilens Config"=w973) -> (w974:T15)
          }
          frame "Open" {
            n317 = Variant To Data(error in=w984, type=FALSE, Variant=w983) -> (data=w981:bool, error out=w985:errorcluster)
            n318 = Bundle By Name(cluster=w986, "Open"=w981) -> (w982:T15)
          }
        }
      }
      frame "Macro: Exit" {
        n319 = Unbundle By Name(w992) -> ("Digilens Config.IO Config.DAQDevices"=w993:T7[])
        n320 = call "DCON Action Engine.vi"("Action"=DCON_Action_Engine-States."Close", "DAQDevices"=w993, "error in (no error)"=w988, "IO In"=w990) -> ("error out"=w989:errorcluster, "IO Out"=w991:refnum<class "IO.lvclass">)  [unwired: 4 in, 2 out]
        n321 = Bundle By Name(cluster=w992, "Open"=FALSE) -> (w996:T15)
        n322 = call <vilib>:"Clear Errors.vi"("error in (no error)"=w989) -> ("error out"=w987:errorcluster)  [unwired: 5 in, 1 out]
        n323 = call <vilib>:"Add States to Queue using MultiLine String (no vData input).vi"("queue in"=w999, "states in"="Quit", "error in"=w987) -> ("error out"=w997:errorcluster)  [unwired: 10 in, 2 out]
      }
      frame "Quit" {
      }
    }
  }
  n324 = Unbundle By Name(w4) -> ("IOLoopEvents"=w3:refnum<user-event>)
  n325 = call <vilib>:"Clear Errors.vi"("error in (no error)"=w7) -> ("error out"=w6:errorcluster)  [unwired: 5 in, 1 out]
  n326 = Destroy User Event(user event=w3, error in=w6) -> (error out=w1:errorcluster)
  n327 = Merge Errors(w19, w1) -> (→"error out":errorcluster)
  "IO out" <- "IO in"
